vi "MC_7_13a_JW.vi"() -> ()   [LabVIEW 2011]
uses:
  <vilib>/Utility/file.llb/Read From Spreadsheet File (string).vi
  <vilib>/Utility/inputDevices.llb/keyboardAcquire.vi
  <vilib>/Utility/file.llb/Write To Spreadsheet File (DBL).vi
  <vilib>/Utility/file.llb/Write To Spreadsheet File (string).vi
  <vilib>/regexp/Match Regular Expression.xnode
panel:
  out "XY Graph-Lin":cluster{dbl[], dbl[]}[](graph)
  out "Lin Vd":dbl
  out "Lin-Vg Array-Used":dbl[](array[numeric])
  out "Lin Id-Used":dbl[](array[numeric])
  out "Rec: Temp":dbl
  out "Comments":string
  out "Folder Index":dbl caption="Length"
  out "Current \nRecord":string[](array[string])
  out "Transformer \nHeaders":string[](array[string])
  out "Current Device ID":string
  out "Column":string
  out "Row":string
  out "Rec: Concentration":dbl
  out "Rec: Solvent":string
  out "Rec: Method":string
  in  "?":T1(tab)
  out "Rec: Material":string
  in  "Treatment Concentration (mM):":dbl=30.0
  in  "Surface Treatment:":string
  in  "# Drops*:":dbl=inf
  in  "Solution Temp (C):":dbl=55.0
  in  "Relative Humidity (%):":dbl=nan
  in  "Room Temp (F):":dbl=nan
  in  "Time (s):":dbl=80.0
  out "Accel (RPM/s):":dbl
  in  "RPM:":dbl=1000.0
  in  "Wait Time (s):":dbl=10.0
  in  "Sample #:":dbl=1.0
  in  "Fabricator:":string="Jeremy"
  in  "Data File":path
  out "Data Folder":path
  in  "Image Folder":path
  out "Image File":path=path "D:/UserData/Desktop/Jeremy/WFU/Research/Programs/VI mods/Image Not Found.png"
  in  "Ramp (s):":dbl=3.0
  in  "Manuel-Dielectric":bool
  in  "Manuel-Length":bool
  out "Calc: VT-Lin":dbl
  out "New: VT-Lin":dbl
  out "Rec: VT-Lin":dbl caption="VT-Lin" format="%#_3g"
  out "Calc: Trap Density-STS":dbl format="%#_4e"
  out "New: Trap Density-STS":dbl format="%#_4e"
  out "Rec: Trap Density-STS":dbl caption="N-Sat (STS)" format="%#_3e"
  out "Calc: Trap Density-VT":dbl format="%#_4e"
  out "New: Trap Density-VT":dbl format="%#_4e"
  out "Rec: Trap Density-VT":dbl caption="N-Sat (VT)" format="%#_3e"
  out "Calc: Mobility-Lin":dbl format="%#_4e"
  out "New: Mobility-Lin":dbl format="%#_4e"
  out "Rec: Mobility-Lin":dbl caption="Mobility-Lin" format="%#_3e"
  out "Calc: Mobility-Sat":dbl format="%#_4e"
  out "Rec: Length":dbl caption="Length" format="%#_3g"
  out "Rec: Width":dbl caption="Width" format="%#_4g"
  out "Rec: Dielectric (d)":dbl caption="Dielectric (d)" format="%#_3g"
  out "XY Graph":cluster{dbl[], dbl[]}[](graph)
  in  "NumPts":dbl=5.0
  in  "Cancel Button":bool
  in  "Next Button":bool
  in  "Previous Button":bool
  in  "Up Button":bool
  in  "Down Button":bool
  out "Data Name:":string
  in  "Save Changes?":bool
  in  "New: Dielectric":dbl
  in  "New: Length":dbl
  in  "New: Width":dbl
  out "New: Mobility-Sat":dbl format="%#_4e"
  in  "Slide":dbl(slide) step=1.0 scale=-14.3..83.0 scale format="%#_1p"
  in  "Blank Button":bool
  in  "Zoom":i16(slide)=-3 scale=-5.0..5.0
  out "Image Out 2":T2(plugin-control)
  out "Image Out":T2(plugin-control)
  in  "Magnification":u16(ring) items=["5x", "10x", "20x", "50x", "80x"]
  out "Total Width":dbl
  out "Distances":dbl[](array[numeric])
  in  "Undo Button":bool
  in  "Remove Button":bool
  out "Rec: Mobility-Sat":dbl caption="Mobility-Sat" format="%#_3e"
  out "Index":string
  out "Image Name":string
  in  "Export":bool
  out "Calc: VT-Sat":dbl
  out "New: VT-Sat":dbl
  in  "Manual-Width":bool caption="Manual"
  out "XY Graph 2":cluster{dbl[], dbl[]}[](graph)
  in  "Next Button 2":bool
  in  "Previous Button 2":bool
  in  "Slide 2":dbl(slide) step=1.0 scale=-1.0..82.0 scale format="%#_1p"
  out "Calc: STS":dbl
  out "New: STS":dbl
  in  "NumPts 2":dbl=5.0 caption="NumPts"
  out "Rec: VT-Sat":dbl caption="VT-Sat" format="%#_3g"
  out "Rec: STS":dbl caption="STS-Sat" format="%#_3g"
  out "Rec: On/Off":dbl caption="On/Off-Sat" format="%#_3e"
  in  "Save Changes? 2":bool
  in  "Save Changes? 3":bool
  out "Date Recorded":string="Date Recorded" caption="Recorded"
  out "Date Created":string caption="Fabricated"
  out "String":string
  in  "No Image":path=path "D:/UserData/Desktop/Jeremy/WFU/Research/Programs/VI mods/Image Not Found.png"
  in  "Project":path=path "D:/UserData/Desktop/Jeremy/WFU/Research/Programs/Mega Awesome/DeviceData.opj"
  out "Index 2":dbl
  out "Sat Id-Log-Used":dbl[](array[numeric])
  out "Vg Array-Log-Used":dbl[](array[numeric])
  out "ROI Descriptor out":T3 {"Contours"."Type" items=["No Selection", "Point", "Line", "Rectangle", "Oval", "Polygon", "Freehand Region", "Annulus", "Unused2", "Unused3", "Broken Line", "Freehand Line", "Rotated Rectangle"]}
  out "ROI Descriptor":T3 {"Contours"."Type" items=["No Selection", "Point", "Line", "Rectangle", "Oval", "Polygon", "Freehand Region", "Annulus", "Unused2", "Unused3", "Broken Line", "Freehand Line", "Rotated Rectangle"]}
  out "Numeric 3":dbl
  out "Array 6":dbl[][](array[numeric])
  out "Cluster":T4
  out "Array 5":dbl[](array[numeric])
  out "Array 4":dbl[](array[numeric])
  out "Array 3":dbl[](array[numeric])
  out "Numeric 2":dbl
  out "Numeric":dbl
  out "Sat Id-Used":dbl[](array[numeric])
  out "Sat Vg Array-Used":dbl[](array[numeric])
  out "MobVi Index":dbl
  in  "Row Start":dbl=20.0
  # "Data Locations"
  # "Data Location"
  # "Image Location"
  # "Sample Properties"
  # "*     Inf = Full coverage\n   NaN = Unknown or Not Applicable"
  # "Recorded"
  # "Calculated"
  # "Re-Calculated"
  # "Manual"
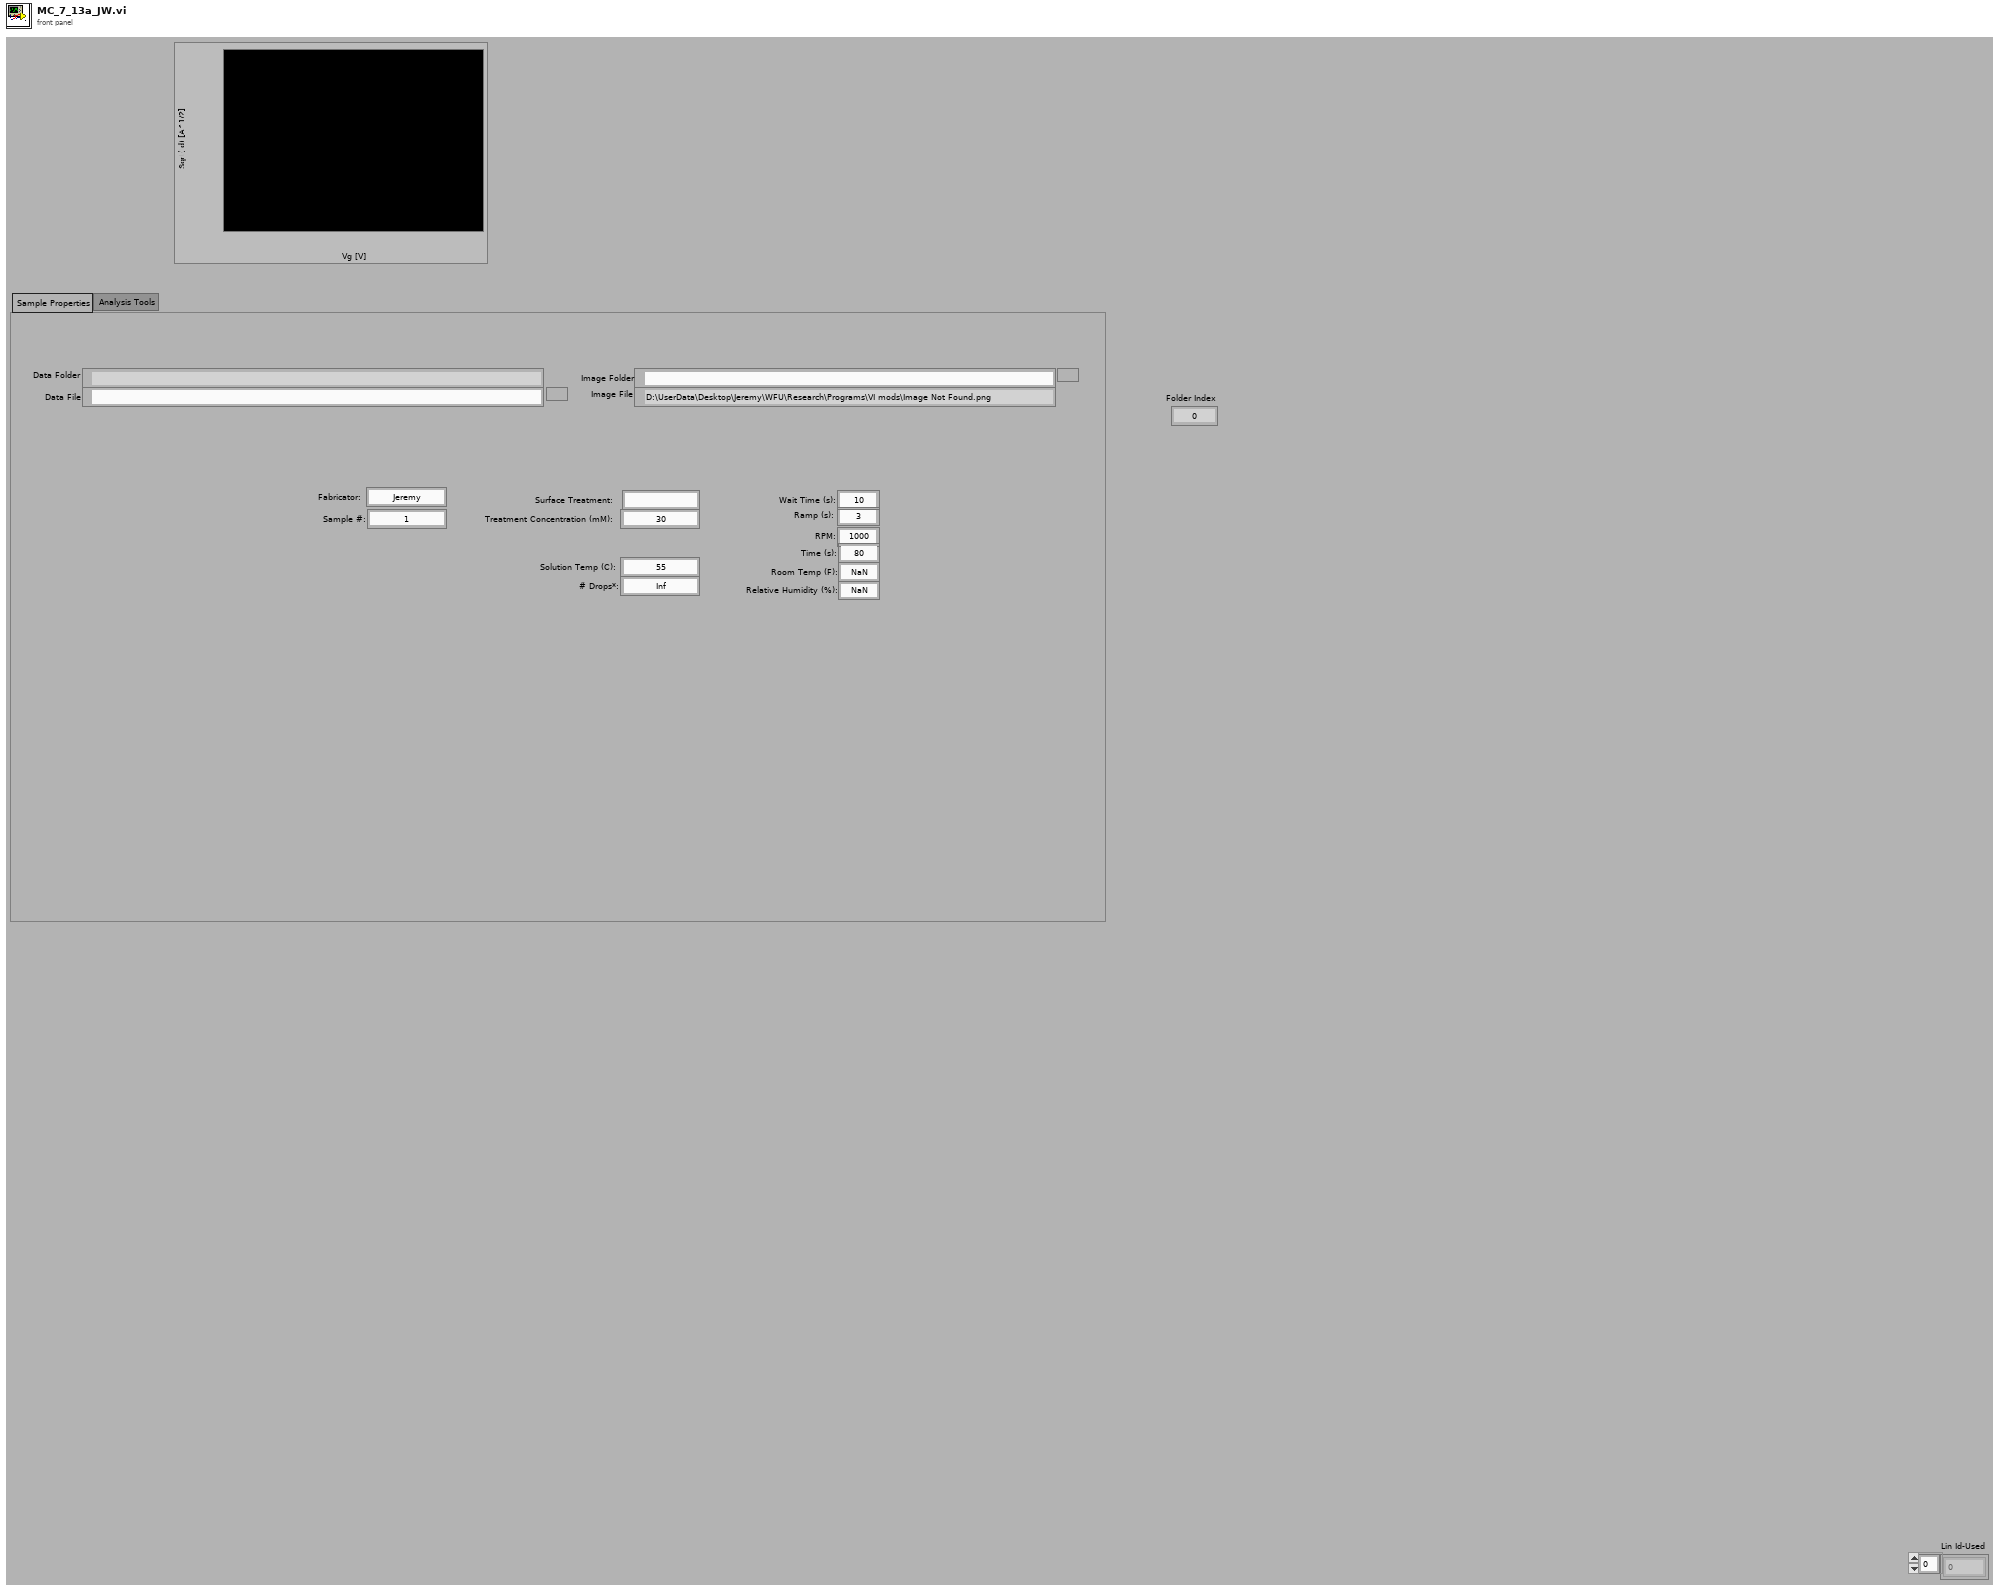
[diagram p1: front panel]
types:
  T1 = enum32{"Sample Properties", "Analysis Tools", "Current Database"}
  T2 = typedef "IMAQ Image.ctl" = refnum<image>
  T3 = typedef "ROI Descriptor" = cluster{"Global Rectangle":i32[], "Contours":cluster{"ID":enum32{"External", "Internal"}, "Type":u32, "Coordinates":i32[]}[]}
  T4 = cluster{"Numeric":dbl, "Numeric 2":dbl, "Numeric 3":dbl, "Numeric 4":dbl}
  T5 = cluster{"Mobility-Sat":dbl, "Moblitity-Lin":dbl, "On/Off":dbl, "Threshold Voltage":dbl, "Onset Voltage":dbl, "STS":dbl, "Trap Density-VT":dbl, "Trap Density-STS":dbl}
  T6 = cluster{"Date Recorded":string, "Index":string, "Length":dbl, "Width":dbl, "Sample Temp":dbl}
  T7 = cluster{"Date Created":string, "Material":string, "Solvent":string, "Concentration":dbl, "Method":string, "Dielectric (nm)":dbl, "Treatment":string, "Comments":string}
  T8 = cluster{"Mobility-Sat":dbl, "Vt-Sat":dbl, "Mobility-Lin":dbl, "Vt-Lin":dbl}
  T9 = cluster{"[0]":cluster{dbl[], dbl[]}, "[1]":cluster{dbl[], dbl[]}, "[2]":cluster{dbl[], dbl[]}, "[3]":cluster{dbl[], dbl[]}, "[4]":cluster{dbl[], dbl[]}, "[5]":cluster{dbl[], dbl[]}, "[6]":cluster{dbl[], dbl[]}, "[7]":cluster{dbl[], dbl[]}, "[8]":cluster{dbl[], dbl[]}}
  T10 = cluster{"Global Rectangle":i32[], "Contours":cluster{"Contour Type":u32, "ROI Type":u32, "Points":i32[]}[]}
  T11 = typedef "LVBoundsTypeDef.ctl" = cluster{"Width":u32, "Height":u32}
  T12 = enum16{"0", "1", "2", "3", "4", "5", "6", "7", "8", "9", "A", "B", "C", "D", "E", "F", "G", "H", "I", "J", "K", "L", "M", "N", "O", "P", "Q", "R", "S", "T", "U", "V", "W", "X", "Y", "Z", "F1", "F2", "F3", "F4", "F5", "F6", "F7", "F8", "F9", "F10", "F11", "F12", "F13", "F14", "F15", "ADD", "BACK", "BACKSLASH", "CAPITAL", "COMMA", "DECIMAL", "DELETE", "DIVIDE", "DOWN", "END", "EQUALS", "ESCAPE", "GRAVE (`)", "HOME", "INSERT", "LBRACKET", "LCONTROL", "LEFT", "L ALT", "LSHIFT", "LWIN", "MINUS", "MULTIPLY", "NEXT", "NUMLOCK", "NUMPAD_0", "NUMPAD_1", "NUMPAD_2", "NUMPAD_3", "NUMPAD_4", "NUMPAD_5", "NUMPAD_6", "NUMPAD_7", "NUMPAD_8", "NUMPAD_9", "PAUSE", "PERIOD", "PRIOR (PG UP)", "RBRACKET", "RCONTROL", "RETURN", "RIGHT", "R ALT", "RSHIFT", "RWIN", "SCROLL", "SEMICOLON", "SLASH", "SPACE", "SUBTRACT", "TAB", "UP", "ENTER (num pad)", "' (quote)"}[]
  T13 = enum16{"0", "1", "2", "3", "4", "5", "6", "7", "8", "9", "A", "B", "C", "D", "E", "F", "G", "H", "I", "J", "K", "L", "M", "N", "O", "P", "Q", "R", "S", "T", "U", "V", "W", "X", "Y", "Z", "F1", "F2", "F3", "F4", "F5", "F6", "F7", "F8", "F9", "F10", "F11", "F12", "F13", "F14", "F15", "ADD", "BACK", "BACKSLASH", "CAPITAL", "COMMA", "DECIMAL", "DELETE", "DIVIDE", "DOWN", "END", "EQUALS", "ESCAPE", "GRAVE (`)", "HOME", "INSERT", "LBRACKET", "LCONTROL", "LEFT", "L ALT", "LSHIFT", "LWIN", "MINUS", "MULTIPLY", "NEXT", "NUMLOCK", "NUMPAD_0", "NUMPAD_1", "NUMPAD_2", "NUMPAD_3", "NUMPAD_4", "NUMPAD_5", "NUMPAD_6", "NUMPAD_7", "NUMPAD_8", "NUMPAD_9", "PAUSE", "PERIOD", "PRIOR (PG UP)", "RBRACKET", "RCONTROL", "RETURN", "RIGHT", "R ALT", "RSHIFT", "RWIN", "SCROLL", "SEMICOLON", "SLASH", "SPACE", "SUBTRACT", "TAB", "UP", "ENTER (num pad)", "' (quote)"}
  T14 = cluster{"Contour Type":u32, "ROI Type":u32, "Points":i32[]}[]
  T15 = cluster{i32[], cluster{"Contour Type":u32, "ROI Type":u32, "Points":i32[]}[]}
  T16 = cluster{string, sgl, bool, bool, bool, bool, bool, bool, i32}
  T17 = cluster{i32, cluster{string, sgl, bool, bool, bool, bool, bool, bool, i32}, i32, i32}
  T18 = cluster{"Contour Type":u32, "ROI Type":u32, "Points":i32[]}
  T19 = cluster{"Points[0]":i32, "Points[1]":i32, "Points[2]":i32, "Points[3]":i32, "Points[4]":i32, "Points[5]":i32, "Points[6]":i32, "Points[7]":i32, "Points[8]":i32}
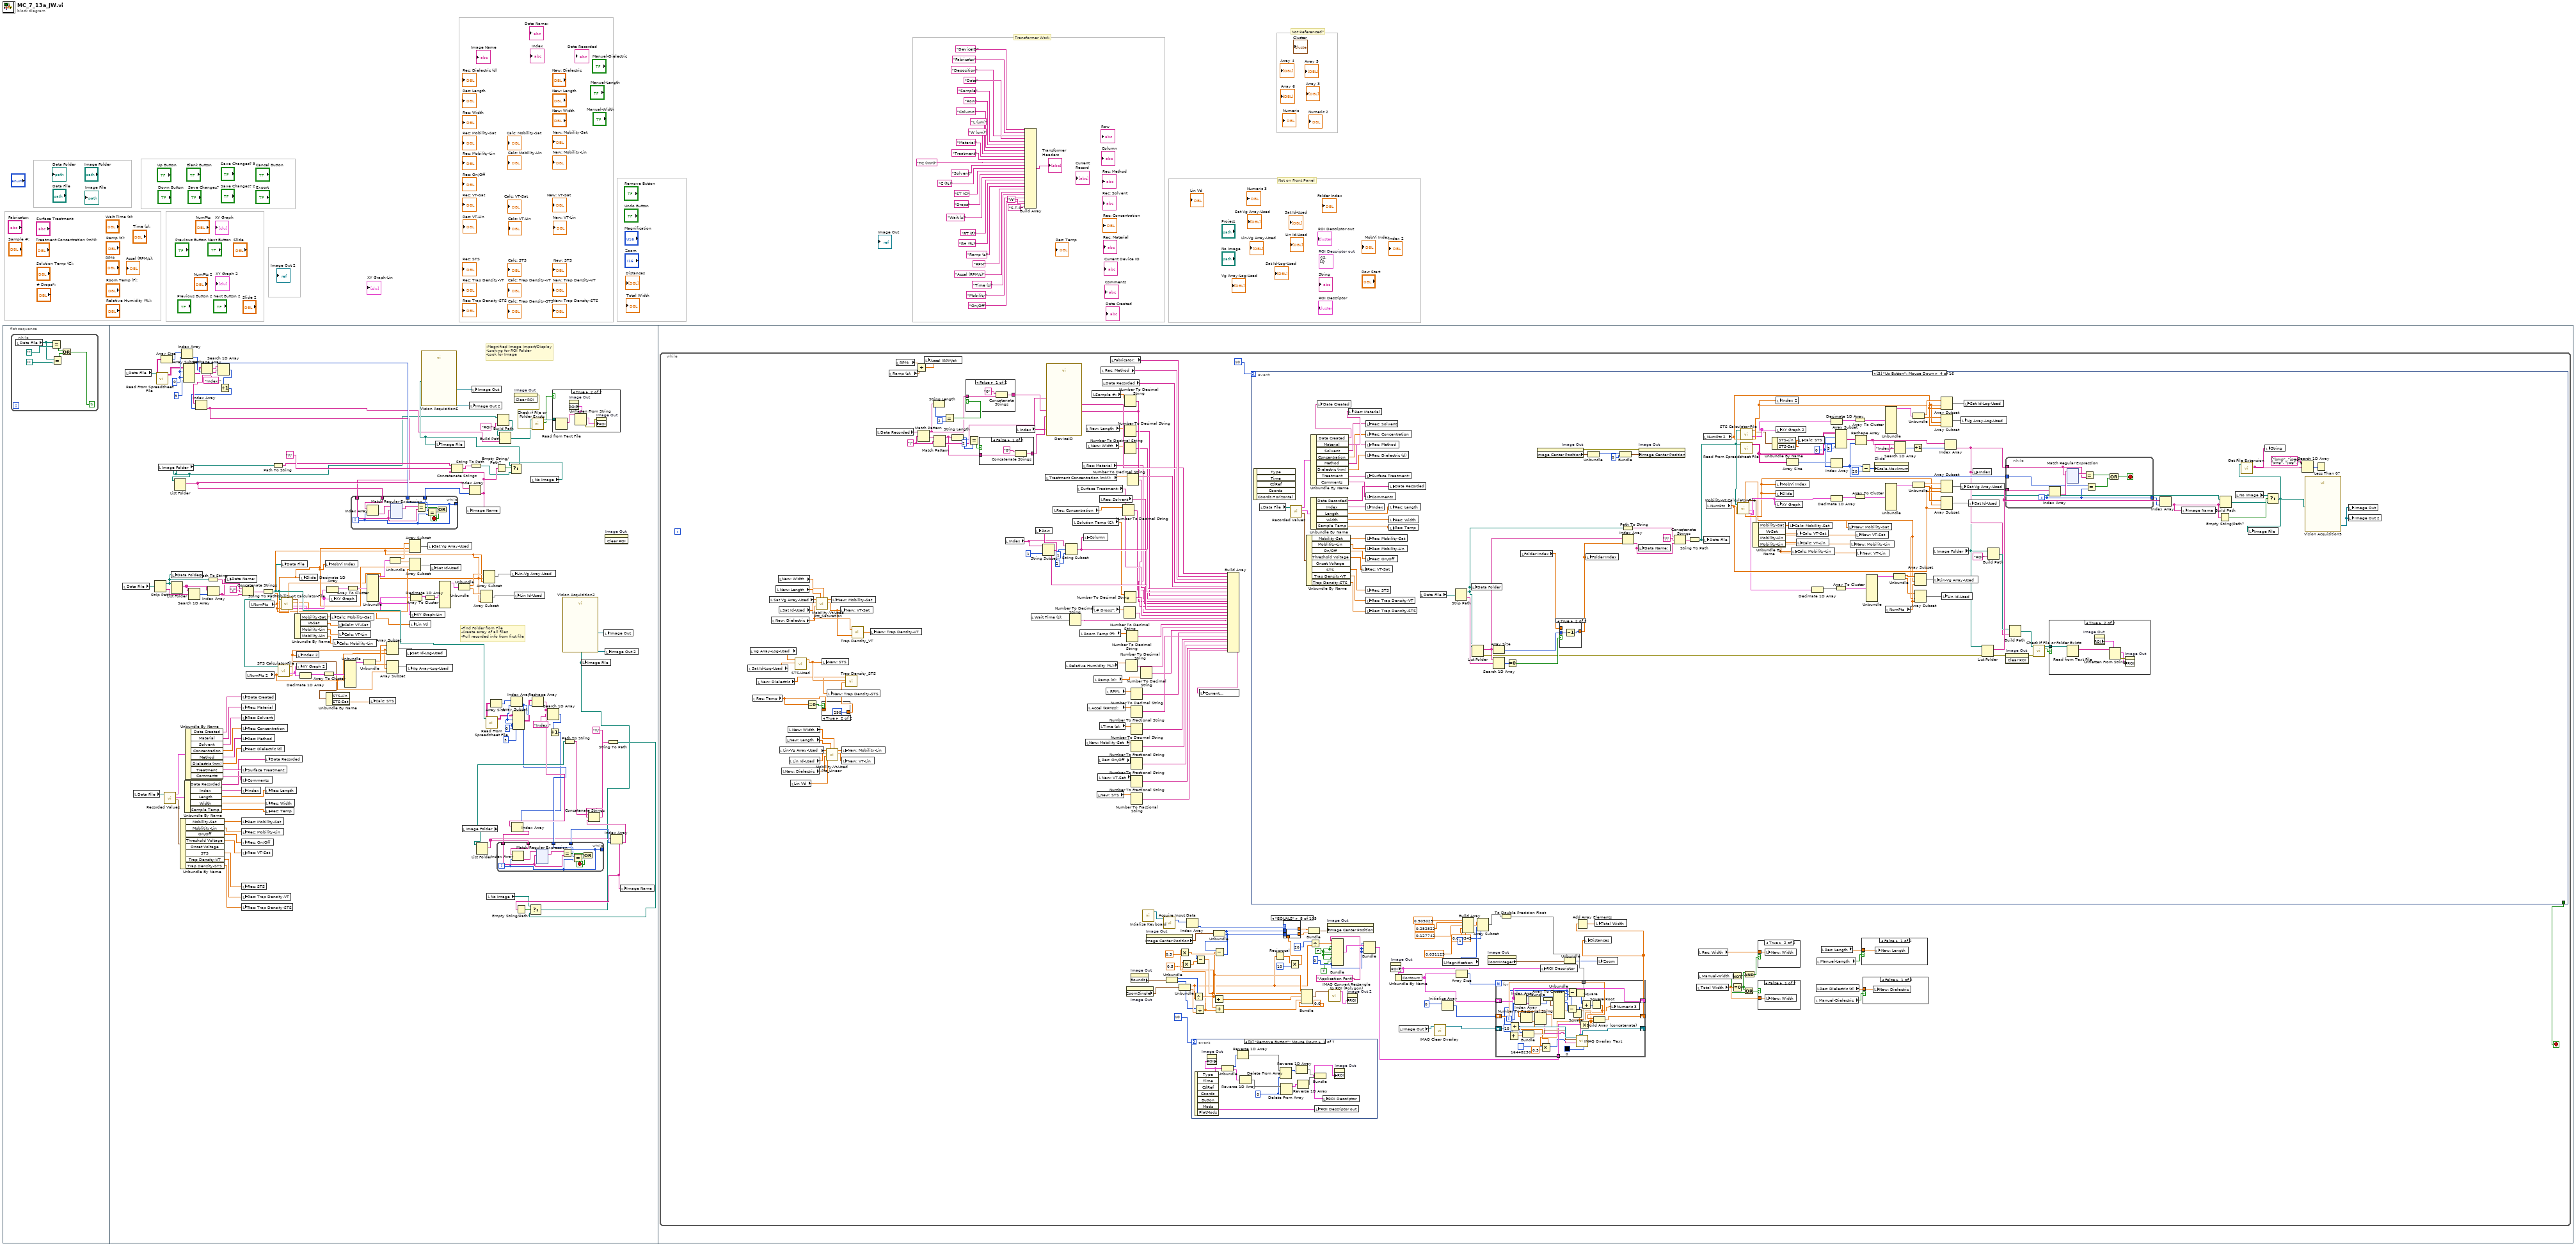
[diagram p0: block diagram]
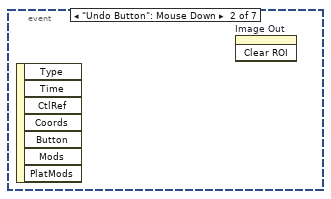
[diagram p10: hidden frame]
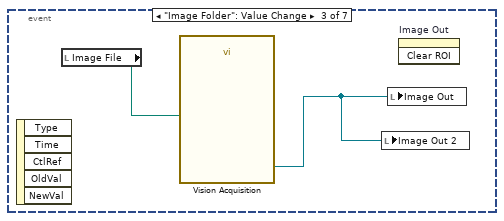
[diagram p11: hidden frame]
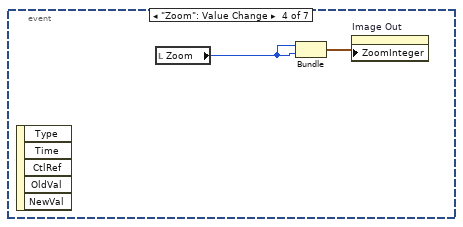
[diagram p12: hidden frame]
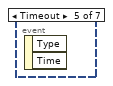
[diagram p13: hidden frame]
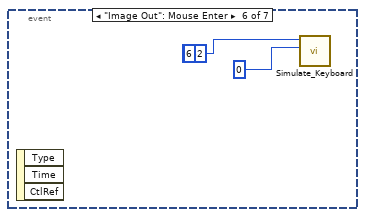
[diagram p14: hidden frame]
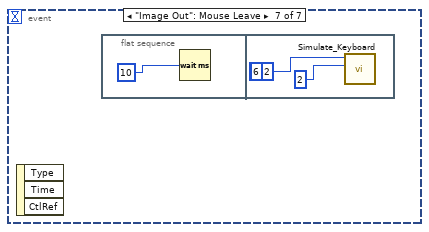
[diagram p15: hidden frame]
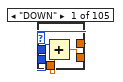
[diagram p16: hidden frame]
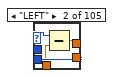
[diagram p17: hidden frame]
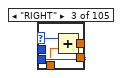
[diagram p18: hidden frame]
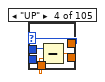
[diagram p19: hidden frame]
diagram:
  (unwired) T3 {"Global Rectangle"=[], "Contours"=[]}  # ROI Descriptor out
  # "Not Referenced?"
  # "Transformer Work"
  # "Not on Front Panel"
  n1 = flat-sequence {
    frame #0 {
      n2 = while {
        stop <- w29 continue-if-true
        n3 = local read "Data File"() -> (w31:path)
        n4 = Equal?(x=w31, y=path "") -> (x = y?=w33:bool)
        n5 = Equal?(x=w31, y=path "") -> (x = y?=w32:bool)
        n6 = Or(x=w33, y=w32) -> (x .or. y?=w29:bool)
      }
    }
    frame #1 {
      w123 = 0
      w147 = 0
      # "-Find Folder from File\n-Create array of all files\n-Pull recorded info from first file"
      # "-Magnified Image Import/Display\n-Looking for ROI Folder\n-Look for Image"
      n7 = local read "Data File"() -> (w127:path)
      n8 = local read "Data File"() -> (w142:path)
      n9 = local read "Data File"() -> (w82:path)
      n10 = Strip Path(path=w127) -> (stripped path=w128:path, name=w114:string)
      n11 = call-poly <vilib>:"Read From Spreadsheet File.vi"("file path (dialog if empty)"=w142) -> ("all rows"=w145:string[][])  [unwired: 6 in, 4 out]
      n12 = local read "Image Folder"() -> (w84:path)
      n13 = Array Size(array=w145) -> (size(s)=w146:i32[])
      n14 = call "Recorded Values.vi"("Path"=w82) -> ("Recorded Char"=w80:T5, "Recorded Prop"=w79:T6, "Fabrication Prop"=w81:T7)  [unwired: 8 in]
      n15 = local write "Data Folder"(w128) -> ()
      n16 = List Folder(path=w128) -> (filenames=w118:string[])  [unwired: 3 in, 3 out]
      n17 = List Folder(path=w84) -> (filenames=w151:string[])  [unwired: 3 in, 3 out]
      n18 = Unbundle By Name(w80) -> ("Mobility-Sat"=w66:dbl, "Moblitity-Lin"=w65:dbl, "On/Off"=w64:dbl, "Threshold Voltage"=w63:dbl, "STS"=w62:dbl, "Trap Density-VT"=w61:dbl, "Trap Density-STS"=w60:dbl)  [unwired: 1 out]
      n19 = Index Array(array=w146, index=w147) -> (element=w153:i32)
      n20 = Array Subset(array=w145, index (row)=w147, index (col)=w147, length (col)=3) -> (w144:string[][])  [unwired: 1 in]
      n21 = Unbundle By Name(w79) -> ("Date Recorded"=w71:string, "Index"=w70:string, "Length"=w69:dbl, "Width"=w68:dbl, "Sample Temp"=w67:dbl)
      n22 = Unbundle By Name(w81) -> ("Date Created"=w59:string, "Material"=w78:string, "Solvent"=w77:string, "Concentration"=w76:dbl, "Method"=w75:string, "Dielectric (nm)"=w74:dbl, "Treatment"=w73:string, "Comments"=w72:string)
      n23 = Search 1D Array(1D array=w118, element=w114) -> (index of element=w117:i32)  [unwired: 1 in]
      n24 = Reshape Array(w144, w153) -> (w158:string[])
      n25 = Path To String(path=w128) -> (string=w113:string)
      n26 = Index Array(array=w118, index=w117) -> (element=w83:string)
      n27 = Search 1D Array(1D array=w158, element="Index:") -> (index of element=w150:i32)  [unwired: 1 in]
      n28 = Increment(x=w150) -> (x+1=w149:i32)
      n29 = Index Array(array=w158, index=w149) -> (element=w85:string)
      n30 = local write "Data Name:"(w83) -> ()
      n31 = local write "Date Created"(w59) -> ()
      n32 = local write "Rec: Material"(w78) -> ()
      n33 = local write "Rec: Solvent"(w77) -> ()
      n34 = local write "Rec: Concentration"(w76) -> ()
      n35 = local write "Rec: Method"(w75) -> ()
      n36 = local write "Rec: Dielectric (d)"(w74) -> ()
      n37 = local write "Surface Treatment:"(w73) -> ()
      n38 = local write "Comments"(w72) -> ()
      n39 = local write "Index"(w70) -> ()
      n40 = local write "Rec: Mobility-Sat"(w66) -> ()
      n41 = local write "Rec: Mobility-Lin"(w65) -> ()
      n42 = local write "Rec: On/Off"(w64) -> ()
      n43 = local write "Rec: VT-Sat"(w63) -> ()
      n44 = local write "Rec: STS"(w62) -> ()
      n45 = local write "Rec: Trap Density-VT"(w61) -> ()
      n46 = local write "Rec: Trap Density-STS"(w60) -> ()
      n47 = Concatenate Strings(w113, "\\", w83) -> (w115:string)
      n48 = local read "NumPts 2"() -> (w50:dbl)
      n49 = local read "NumPts"() -> (w40:dbl)
      n50 = String To Path(string=w115) -> (path=w58:path)
      n51 = local write "Date Recorded"(w71) -> ()
      n52 = local write "Rec: Length"(w69) -> ()
      n53 = local write "Rec: Width"(w68) -> ()
      n54 = local write "Rec: Temp"(w67) -> ()
      n55 = Path To String(path=w84) -> (string=w155:string)
      n56 = call "STS Calculator-File.vi"("NumPts"=w50, "Path"=w58) -> ("STS Index-Sat"=w48:dbl, "XY Graph-Sat"=w49:cluster{dbl[], dbl[]}[], "Ouput"=w47:cluster{"STS-Sat":dbl, "STS-Lin":dbl})  [unwired: 5 in, 2 out]
      n57 = local write "Data File"(w58) -> ()
      n58 = call "Mobility-Vt Calculator-File.vi"("NumPts"=w40, "Path"=w58) -> ("XY Graph-Sat"=w52:cluster{dbl[], dbl[]}[], "XY Graph-Lin"=w35:cluster{dbl[], dbl[]}[], "Lin Vd"=w36:dbl, "Output"=w53:T8, "Index-Sat"=w51:dbl, "Index-Lin"=w39:dbl)  [unwired: 4 in]
      n59 = Unbundle By Name(w53) -> ("Mobility-Sat"=w57:dbl, "Vt-Sat"=w56:dbl, "Mobility-Lin"=w55:dbl, "Mobility-Lin"=w54:dbl)
      n60 = local write "Index 2"(w48) -> ()
      n61 = local write "XY Graph 2"(w49) -> ()
      n62 = local write "Slide"(w51) -> ()
      n63 = Decimate 1D Array(w49) -> (w105:cluster{dbl[], dbl[]}[])  [unwired: 1 out]
      n64 = Array To Cluster(array=w105) -> (cluster=w107:T9)
      n65 = local write "MobVi Index"(w51) -> ()
      n66 = Unbundle By Name(w47) -> ("STS-Sat"=w46:dbl)  [unwired: 1 out]
      n67 = Decimate 1D Array(w52) -> (w141:cluster{dbl[], dbl[]}[])  [unwired: 1 out]
      n68 = local write "XY Graph"(w52) -> ()
      n69 = local write "Calc: Mobility-Sat"(w57) -> ()
      n70 = local write "Calc: Mobility-Lin"(w54) -> ()
      n71 = local write "Calc: VT-Sat"(w56) -> ()
      n72 = local write "Calc: VT-Lin"(w55) -> ()
      n73 = Unbundle(w107) -> ("[0]"=w106:cluster{dbl[], dbl[]})  [unwired: 8 out]
      n74 = Array To Cluster(array=w141) -> (cluster=w139:T9)
      n75 = while {
        tunnel: w151 -> [w291]
        tunnel: w85 -> [w289]
        tunnel: [w288] -> _
        tunnel: [w288] -> w152
        tunnel: w153 -> [w287]
        i -> [w288]
        stop <- w284 stop-if-true
        n76 = Index Array(array=w291, index=w288) -> (element=w292:string)
        n77 = xnode "Match Regular Expression"("input string"=w292, "regular expression"=w289) -> ("whole match"=w290:string)  [unwired: 4 in, 4 out]
        n78 = Equal?(x=w290, y=w289) -> (x = y?=w286:bool)
        n79 = Equal?(x=w287, y=w288) -> (x = y?=w285:bool)
        n80 = Or(x=w286, y=w285) -> (x .or. y?=w284:bool)
      }
      n81 = Unbundle(w106) -> (w103:dbl[], w102:dbl[])
      n82 = Unbundle(w139) -> ("[0]"=w140:cluster{dbl[], dbl[]})  [unwired: 8 out]
      n83 = local write "Calc: STS"(w46) -> ()
      n84 = Array Subset(array=w103, index=w48, length=w50) -> (w110:dbl[])
      n85 = Array Subset(array=w102, index=w48, length=w50) -> (w109:dbl[])
      n86 = Unbundle(w140) -> (w104:dbl[], w108:dbl[])
      n87 = local write "Sat Id-Log-Used"(w110) -> ()
      n88 = local write "Vg Array-Log-Used"(w109) -> ()
      n89 = Array Subset(array=w104, index=w51, length=w40) -> (w111:dbl[])
      n90 = Array Subset(array=w108, index=w51, length=w40) -> (w112:dbl[])
      n91 = local write "Lin Vd"(w36) -> ()
      n92 = Decimate 1D Array(w35) -> (w45:cluster{dbl[], dbl[]}[])  [unwired: 1 out]
      n93 = local write "XY Graph-Lin"(w35) -> ()
      n94 = Array To Cluster(array=w45) -> (cluster=w44:T9)
      n95 = local write "Sat Vg Array-Used"(w111) -> ()
      n96 = local write "Sat Id-Used"(w112) -> ()
      n97 = Unbundle(w44) -> ("[0]"=w43:cluster{dbl[], dbl[]})  [unwired: 8 out]
      n98 = Unbundle(w43) -> (w42:dbl[], w41:dbl[])
      n99 = local read "Image Folder"() -> (w134:path)
      n100 = Index Array(array=w151, index=w152) -> (element=w101:string)
      n101 = Concatenate Strings(w155, "\\", w101) -> (w156:string)
      n102 = local write "Image Name"(w101) -> ()
      n103 = String To Path(string=w156) -> (path=w99:path)
      n104 = List Folder(path=w134) -> (filenames=w130:string[])  [unwired: 3 in, 3 out]
      n105 = Array Subset(array=w41, index=w39, length=w40) -> (w37:dbl[])
      n106 = Array Subset(array=w42, index=w39, length=w40) -> (w38:dbl[])
      n107 = call-poly <vilib>:"Read From Spreadsheet File.vi"("file path (dialog if empty)"=w58) -> ("all rows"=w121:string[][])  [unwired: 6 in, 4 out]
      n108 = local read "No Image"() -> (w93:path)
      n109 = Array Size(array=w121) -> (size(s)=w122:i32[])
      n110 = Empty String/Path?(string/path=w101) -> (empty?=w100:bool)
      n111 = Build Path(base path=w84, name or relative path="ROI") -> (appended path=w87:path)
      n112 = Build Path(base path=w87, name or relative path=w85) -> (appended path=w86:path)
      n113 = Index Array(array=w122, index=w123) -> (element=w133:i32)
      n114 = local write "Lin-Vg Array-Used"(w38) -> ()
      n115 = Array Subset(array=w121, index (row)=w123, index (col)=w123, length (col)=3) -> (w120:string[][])  [unwired: 1 in]
      n116 = local write "Lin Id-Used"(w37) -> ()
      n117 = invoke on="Image Out" class="ImageControl" method="Clear ROI"() -> (error out=w91:errorcluster)  [unwired: 3 in, 2 out]
      n118 = local read "No Image"() -> (w92:path)
      n119 = Select(t=w92, s=w100, f=w99) -> (s? t:f=w98:path)
      n120 = call "Vision Acquisition6"("Image Path"=w98) -> ("Image Out"=w154:T2)  [unwired: 25 in, 1 out]
      n121 = local write "Image File"(w98) -> ()
      n122 = local write "Image Out 2"(w154) -> ()
      n123 = local write "Image Out"(w154) -> ()
      n124 = call <vilib>:"Check if File or Folder Exists.vi"("error in (no error)"=w91, "path"=w86) -> ("file or folder exists?"=w89:bool, "dup path"=w90:path)  [unwired: 7 in, 1 out]
      n125 = Reshape Array(w120, w133) -> (w138:string[])
      n126 = Search 1D Array(1D array=w138, element="Index:") -> (index of element=w126:i32)  [unwired: 1 in]
      n127 = Increment(x=w126) -> (x+1=w125:i32)
      n128 = Index Array(array=w138, index=w125) -> (element=w131:string)
      n129 = while {
        tunnel: w130 -> [w171]
        tunnel: w131 -> [w169]
        tunnel: [w168] -> _
        tunnel: [w168] -> w132
        tunnel: w133 -> [w167]
        i -> [w168]
        stop <- w164 stop-if-true
        n130 = Index Array(array=w171, index=w168) -> (element=w172:string)
        n131 = xnode "Match Regular Expression"("input string"=w172, "regular expression"=w169) -> ("whole match"=w170:string)  [unwired: 4 in, 4 out]
        n132 = Equal?(x=w170, y=w169) -> (x = y?=w166:bool)
        n133 = Equal?(x=w167, y=w168) -> (x = y?=w165:bool)
        n134 = Or(x=w166, y=w165) -> (x .or. y?=w164:bool)
      }
      n135 = case shown="True" w89 {
        tunnel: w90 -> [_ w159]
        frame False {
        }
        frame True {
          n136 = Read from Text File(file (use dialog)=w159) -> (text=w163:string)  [unwired: 3 in, 3 out]
          n137 = property on="Image Out" class="ImageControl"() -> ("ROI"=w160:T10)  [unwired: 2 in, 2 out]
          n138 = Unflatten From String(type=w160, binary string=w163) -> (value=w161:T10, error out=w162:errorcluster)  [unwired: 3 in, 1 out]
          n139 = property on="Image Out" class="ImageControl"(error in=w162, "ROI"=w161) -> ()  [unwired: 1 in, 2 out]
        }
      }
      n140 = Path To String(path=w134) -> (string=w135:string)
      n141 = invoke on="Image Out" class="ImageControl" method="Clear ROI"() -> ()  [unwired: 3 in, 3 out]
      n142 = Index Array(array=w130, index=w132) -> (element=w96:string)
      n143 = Empty String/Path?(string/path=w96) -> (empty?=w97:bool)
      n144 = Concatenate Strings(w135, "\\", w96) -> (w136:string)
      n145 = String To Path(string=w136) -> (path=w95:path)
      n146 = Select(t=w93, s=w97, f=w95) -> (s? t:f=w94:path)
      n147 = call "Vision Acquisition2"("Image Path"=w94) -> ("Image Out"=w129:T2)  [unwired: 25 in, 1 out]
      n148 = local write "Image File"(w94) -> ()
      n149 = local write "Image Out"(w129) -> ()
      n150 = local write "Image Out 2"(w129) -> ()
      n151 = local write "Image Name"(w96) -> ()
    }
    frame #2 {
      n152 = while {
        stop <- w569 stop-if-true
        w465 = "/"
        w519 = FALSE
        w517 = 0
        n153 = local read "Sat Id-Log-Used"() -> (w422:dbl[])
        n154 = local read "Vg Array-Log-Used"() -> (w421:dbl[])
        n155 = local read "Rec: Temp"() -> (w411:dbl)
        n156 = local read "New: Dielectric"() -> (w408:dbl)
        n157 = local read "Sat Vg Array-Used"() -> (w424:dbl[])
        n158 = local read "New: Dielectric"() -> (w405:dbl)
        n159 = local read "New: Length"() -> (w425:dbl)
        n160 = local read "New: Width"() -> (w427:dbl)
        n161 = local read "Sat Id-Used"() -> (w423:dbl[])
        n162 = local read "Lin-Vg Array-Used"() -> (w418:dbl[])
        n163 = local read "New: Dielectric"() -> (w415:dbl)
        n164 = local read "New: Length"() -> (w417:dbl)
        n165 = local read "New: Width"() -> (w414:dbl)
        n166 = local read "Lin Id-Used"() -> (w419:dbl[])
        n167 = local read "Lin Vd"() -> (w413:dbl)
        n168 = call "STS-Used.vi"("Id Used"=w422, "Vg-Used"=w421) -> ("STS"=w412:dbl)  [unwired: 9 in]
        n169 = Equal To 0?(x=w411) -> (x = 0?=w410:bool)
        n170 = call "Mobility-Vt-Used Pts_Saturation.vi"("Width"=w427, "Length"=w425, "Dielectric (d)"=w405, "Sat Id Used"=w423, "Vg Used"=w424) -> ("Vt"=w406:dbl, "Mobility"=w426:dbl)  [unwired: 4 in, 1 out]
        n171 = local write "New: STS"(w412) -> ()
        n172 = case shown="True" w410 {
          tunnel: [w570 290] -> w409
          tunnel: w411 -> [w570 _]
          frame False {
          }
          frame True {
          }
        }
        n173 = call "Mobility-Vt-Used Pts_Linear.vi"("Width"=w414, "Length"=w417, "Vd"=w413, "Dielectric (d)"=w415, "Sat Id Used"=w419, "Vg Used"=w418) -> ("Vt"=w420:dbl, "Mobility"=w416:dbl)  [unwired: 3 in, 1 out]
        n174 = local write "New: Mobility-Sat"(w426) -> ()
        n175 = local write "New: VT-Sat"(w406) -> ()
        n176 = local write "New: Mobility-Lin"(w416) -> ()
        n177 = local write "New: VT-Lin"(w420) -> ()
        n178 = call "Trap Density_STS.vi"("Temp (T) [K]"=w409, "S.T.S. (S)"=w412, "Dielectric"=w408) -> ("Trap Density (N)"=w407:dbl)  [unwired: 8 in]
        n179 = local write "New: Trap Density-STS"(w407) -> ()
        n180 = call "Trap Density_VT.vi"("VT"=w406, "Dielectric"=w405) -> ("Trap Density-VT"=w404:dbl)
        n181 = local write "New: Trap Density-VT"(w404) -> ()
        n182 = local read "Date Recorded"() -> (w468:string)
        n183 = local read "Ramp (s):"() -> (w435:dbl)
        n184 = local read "RPM:"() -> (w436:dbl)
        n185 = Divide(x=w436, y=w435) -> (x/y=w434:dbl)
        n186 = Match Pattern(string=w468, regular expression=w465) -> (before substring=w459:string, after substring=w466:string)  [unwired: 1 in, 2 out]
        n187 = local write "Accel (RPM/s):"(w434) -> ()
        n188 = String Length(string=w459) -> (length=w462:i32)
        n189 = Match Pattern(string=w466, regular expression=w465) -> (before substring=w453:string, after substring=w464:string)  [unwired: 1 in, 2 out]
        n190 = Equal?(x=w462, y=2) -> (x = y?=w460:bool)
        n191 = String Length(string=w453) -> (length=w455:i32)
        n192 = case shown="False" w460 {
          tunnel: w459 -> [w579 w581]
          tunnel: [w578 w581] -> w458
          frame False {
            n193 = Concatenate Strings("0", w579) -> (w578:string)
          }
          frame True {
          }
        }
        n194 = Equal?(x=w455, y=2) -> (x = y?=w457:bool)
        n195 = case shown="False" w457 {
          tunnel: w453 -> [w575 w577]
          tunnel: [w574 w577] -> w454
          frame False {
            n196 = Concatenate Strings("0", w575) -> (w574:string)
          }
          frame True {
          }
        }
        n197 = local read "Index"() -> (w438:string)
        n198 = local read "Index"() -> (w452:string)
        n199 = local read "Wait Time (s):"() -> (w498:dbl)
        n200 = String Subset(string=w438, length (rest)=1) -> (substring=w493:string)  [unwired: 1 in]
        n201 = local write "Row"(w493) -> ()
        n202 = local read "Treatment Concentration (mM):"() -> (w446:dbl)
        n203 = local read "Rec: Concentration"() -> (w433:dbl)
        n204 = local read "Relative Humidity (%):"() -> (w443:dbl)
        n205 = String Subset(string=w438, offset (0)=1, length (rest)=2) -> (substring=w494:string)
        n206 = Number To Decimal String(number=w498) -> (decimal integer string=w499:string)  [unwired: 1 in]
        n207 = local read "Solution Temp (C):"() -> (w487:dbl)
        n208 = local read "Surface Treatment:"() -> (w445:string)
        n209 = local read "Room Temp (F):"() -> (w491:dbl)
        n210 = local read "Rec: Material"() -> (w441:string)
        n211 = local write "Column"(w494) -> ()
        n212 = local read "New: Mobility-Sat"() -> (w480:dbl)
        n213 = local read "New: Length"() -> (w451:dbl)
        n214 = local read "New: Width"() -> (w450:dbl)
        n215 = local read "Accel (RPM/s):"() -> (w478:dbl)
        n216 = local read "Sample #:"() -> (w470:dbl)
        n217 = local read "# Drops*:"() -> (w488:dbl)
        n218 = local read "Ramp (s):"() -> (w496:dbl)
        n219 = local read "New: STS"() -> (w472:dbl)
        n220 = local read "New: VT-Sat"() -> (w474:dbl)
        n221 = local read "Rec: On/Off"() -> (w476:dbl)
        n222 = local read "Rec: Solvent"() -> (w447:string)
        n223 = local read "Time (s):"() -> (w483:dbl)
        n224 = local read "Rec: Method"() -> (w471:string)
        n225 = local read "Date Recorded"() -> (w467:string)
        n226 = local read "RPM:"() -> (w484:dbl)
        n227 = local read "Fabricator:"() -> (w492:string)
        n228 = Number To Decimal String(number=w433) -> (decimal integer string=w432:string)  [unwired: 1 in]
        n229 = Number To Decimal String(number=w488) -> (decimal integer string=w489:string)  [unwired: 1 in]
        n230 = Number To Decimal String(number=w470) -> (decimal integer string=w463:string)  [unwired: 1 in]
        n231 = call "DeviceID"("Sample"=w463, "Year"=w464, "Month"=w458, "Day"=w454, "Index"=w452) -> ("Result"=w469:string)  [unwired: 9 in, 1 out]
        n232 = Number To Decimal String(number=w451) -> (decimal integer string=w449:string)  [unwired: 1 in]
        n233 = Number To Decimal String(number=w450) -> (decimal integer string=w448:string)  [unwired: 1 in]
        n234 = Number To Decimal String(number=w487) -> (decimal integer string=w486:string)  [unwired: 1 in]
        n235 = Number To Decimal String(number=w443) -> (decimal integer string=w442:string)  [unwired: 1 in]
        n236 = Number To Decimal String(number=w491) -> (decimal integer string=w490:string)  [unwired: 1 in]
        n237 = property on="Image Out" class="ImageControl"() -> ("ZoomSingle"=w537:cluster{"X":sgl, "Y":sgl})  [unwired: 2 in, 2 out]
        n238 = Number To Decimal String(number=w446) -> (decimal integer string=w444:string)  [unwired: 1 in]
        n239 = property on="Image Out" class="ImageControl"() -> ("Bounds"=w538:T11)  [unwired: 2 in, 2 out]
        n240 = Number To Decimal String(number=w484) -> (decimal integer string=w485:string)  [unwired: 1 in]
        n241 = Number To Fractional String(number=w478) -> (F-format string=w479:string)  [unwired: 3 in]
        n242 = Number To Decimal String(number=w483) -> (decimal integer string=w482:string)  [unwired: 1 in]
        n243 = Number To Fractional String(number=w480) -> (F-format string=w481:string)  [unwired: 3 in]
        n244 = Number To Fractional String(number=w476) -> (F-format string=w477:string)  [unwired: 3 in]
        n245 = Number To Fractional String(number=w474) -> (F-format string=w475:string)  [unwired: 3 in]
        n246 = Number To Fractional String(number=w472) -> (F-format string=w473:string)  [unwired: 3 in]
        n247 = Number To Decimal String(number=w496) -> (decimal integer string=w497:string)  [unwired: 1 in]
        n248 = call <vilib>:"Intialize Keyboard.vi"() -> ("device ID"=w549:refnum<k1>)  [unwired: 10 in, 1 out]
        n249 = property on="Image Out" class="ImageControl"() -> ("Image Center Position"=w544:cluster{"X":u32, "Y":u32})  [unwired: 2 in, 2 out]
        n250 = call-poly <vilib>:"Acquire Input Data.vi"("device ID"=w549) -> ("keys pressed"=w548:T12)  [unwired: 16 in, 2 out]
        n251 = Unbundle(w538) -> ("Width"=w535:u32, "Height"=w534:u32)
        n252 = Unbundle(w537) -> ("X"=w512:sgl, "Y"=w536:sgl)
        n253 = Index Array(array=w548) -> (element=w552:T13)  [unwired: 1 in]
        n254 = event shown="[0] \"Remove Button\": Mouse Down" {
          selector: _ -> [_ _ _ _ _ _ _]
          dyn-events: _ -> [_ _ _ _ _ _ _]
          timeout: 10 -> [_ _ _ _ _ _ _]
          event "Remove Button": Mouse Down {
            w586 = 0
            n255 = event-data() -> ()  [unwired: 1 in, 7 out]
            n256 = property on="Image Out" class="ImageControl"() -> ("ROI"=w584:T10)  [unwired: 2 in, 2 out]
            n257 = Unbundle(w584) -> ("Global Rectangle"=w587:i32[], "Contours"=w589:T14)
            n258 = Reverse 1D Array(array=w587) -> (reversed array=w588:i32[])
            n259 = Reverse 1D Array(array=w589) -> (reversed array=w590:T14)
            n260 = Delete From Array(array=w588, index=w586) -> (array with subset deleted=w591:i32[])  [unwired: 1 in, 1 out]
            n261 = Delete From Array(array=w590, index=w586) -> (array with subset deleted=w592:T14)  [unwired: 1 in, 1 out]
            n262 = Reverse 1D Array(array=w591) -> (reversed array=w593:i32[])
            n263 = Reverse 1D Array(array=w592) -> (reversed array=w594:T14)
            n264 = Bundle(w593, w594) -> (w585:T15)  [unwired: 1 in]
            n265 = local write "ROI Descriptor out"(w584) -> ()
            n266 = local write "ROI Descriptor"(w585) -> ()
            n267 = property on="Image Out" class="ImageControl"("ROI"=w585) -> ()  [unwired: 2 in, 2 out]
          }
          event "Undo Button": Mouse Down {
            n268 = event-data() -> ()  [unwired: 1 in, 7 out]
            n269 = invoke on="Image Out" class="ImageControl" method="Clear ROI"() -> ()  [unwired: 3 in, 3 out]
          }
          event "Image Folder": Value Change {
            n270 = event-data() -> ()  [unwired: 1 in, 5 out]
            n271 = local read "Image File"() -> (w596:path)
            n272 = call "Vision Acquisition"("Image Path"=w596) -> ("Image Out"=w595:T2)  [unwired: 25 in, 1 out]
            n273 = local write "Image Out 2"(w595) -> ()
            n274 = local write "Image Out"(w595) -> ()
            n275 = invoke on="Image Out" class="ImageControl" method="Clear ROI"() -> ()  [unwired: 3 in, 3 out]
          }
          event "Zoom": Value Change {
            n276 = event-data() -> ()  [unwired: 1 in, 5 out]
            n277 = local read "Zoom"() -> (w597:i16)
            n278 = Bundle("Zoom"=w597, "Zoom"=w597) -> (w598:cluster{"Zoom":i16, "Zoom":i16})  [unwired: 1 in]
            n279 = property on="Image Out" class="ImageControl"("ZoomInteger"=w598) -> ()  [unwired: 2 in, 2 out]
          }
          event Timeout {
            n280 = event-data() -> ()  [unwired: 1 in, 2 out]
          }
          event "Image Out": Mouse Enter {
            (unwired) 6
            n281 = event-data() -> ()  [unwired: 1 in, 3 out]
            n282 = call "Simulate_Keyboard.vi"("Action"=0, "Virtual Key"=162) -> ()  [unwired: 7 in, 1 out]
          }
          event "Image Out": Mouse Leave {
            n283 = event-data() -> ()  [unwired: 1 in, 3 out]
            n284 = flat-sequence {
              frame #0 {
                n285 = Wait (ms)(milliseconds to wait=10) -> ()  [unwired: 1 out]
              }
              frame #1 {
                (unwired) 6
                n286 = call "Simulate_Keyboard.vi"("Action"=2, "Virtual Key"=162) -> ()  [unwired: 7 in, 1 out]
              }
            }
          }
        }
        n287 = Divide(x=w535, y=w512) -> (x/y=w525:sgl)
        n288 = Multiply(x=w525, y=0.5) -> (x*y=w531:dbl)
        n289 = Divide(x=w534, y=w536) -> (x/y=w524:sgl)
        n290 = Multiply(x=w524, y=0.5) -> (x*y=w530:dbl)
        n291 = Unbundle(w544) -> ("X"=w526:u32, "Y"=w527:u32)
        n292 = Subtract(x=w527, y=w530) -> (x-y=w528:dbl)
        n293 = Subtract(x=w526, y=w531) -> (x-y=w529:dbl)
        n294 = Add(x=w529, y=w525) -> (x+y=w543:dbl)
        n295 = Add(x=w528, y=w524) -> (x+y=w542:dbl)
        n296 = Build Array(w469, w492, w471, w467, w463, w493, w494, w449, w448, w441, w445, w444, w447, w432, w486, w489, w499, w490, w442, w497, w485, w479, w482, w481, w477, w475, w473) -> (w495:string[])
        n297 = local write "Current \nRecord"(w495) -> ()
        n298 = event shown="[3] \"Up Button\": Mouse Down" {
          selector: _ -> [_ _ _ _ _ _ _ _ _ _ _ _ _ _ _ _]
          dyn-events: _ -> [_ _ _ _ _ _ _ _ _ _ _ _ _ _ _ _]
          timeout: 10 -> [_ _ _ _ _ _ _ _ _ _ _ _ _ _ _ _]
          tunnel: [_ _ _ _ _ _ _ _ _ _ _ _ _ TRUE _ TRUE] -> w569
          event Timeout {
            n299 = event-data() -> ()  [unwired: 1 in, 2 out]
          }
          event "Down Button": Mouse Down {
            w929 = 0
            n300 = event-data() -> ()  [unwired: 1 in, 7 out]
            n301 = local read "Data File"() -> (w945:path)
            n302 = call "Recorded Values.vi"("Path"=w945) -> ("Recorded Char"=w947:T5, "Recorded Prop"=w948:T6, "Fabrication Prop"=w946:T7)  [unwired: 8 in]
            n303 = Unbundle By Name(w947) -> ("Mobility-Sat"=w961:dbl, "Moblitity-Lin"=w962:dbl, "On/Off"=w963:dbl, "Threshold Voltage"=w964:dbl, "STS"=w965:dbl, "Trap Density-VT"=w966:dbl, "Trap Density-STS"=w967:dbl)  [unwired: 1 out]
            n304 = Unbundle By Name(w946) -> ("Date Created"=w968:string, "Material"=w949:string, "Solvent"=w950:string, "Concentration"=w951:dbl, "Method"=w952:string, "Dielectric (nm)"=w953:dbl, "Treatment"=w954:string, "Comments"=w955:string)
            n305 = Unbundle By Name(w948) -> ("Date Recorded"=w956:string, "Index"=w957:string, "Length"=w958:dbl, "Width"=w959:dbl, "Sample Temp"=w960:dbl)
            n306 = local write "Date Created"(w968) -> ()
            n307 = local write "Rec: VT-Sat"(w964) -> ()
            n308 = local write "Rec: Material"(w949) -> ()
            n309 = local write "Rec: Concentration"(w951) -> ()
            n310 = local write "Rec: Method"(w952) -> ()
            n311 = local write "Rec: Dielectric (d)"(w953) -> ()
            n312 = local write "Surface Treatment:"(w954) -> ()
            n313 = local write "Comments"(w955) -> ()
            n314 = local write "Index"(w957) -> ()
            n315 = local write "Rec: Mobility-Sat"(w961) -> ()
            n316 = local write "Rec: Mobility-Lin"(w962) -> ()
            n317 = local write "Rec: On/Off"(w963) -> ()
            n318 = local write "Rec: STS"(w965) -> ()
            n319 = local write "Rec: Trap Density-VT"(w966) -> ()
            n320 = local write "Rec: Trap Density-STS"(w967) -> ()
            n321 = local write "Rec: Solvent"(w950) -> ()
            n322 = local write "Date Recorded"(w956) -> ()
            n323 = local write "Rec: Length"(w958) -> ()
            n324 = local write "Rec: Width"(w959) -> ()
            n325 = local write "Rec: Temp"(w960) -> ()
            n326 = local read "Data File"() -> (w934:path)
            n327 = Strip Path(path=w934) -> (stripped path=w925:path, name=w943:string)
            n328 = local write "Data Folder"(w925) -> ()
            n329 = List Folder(path=w925) -> (filenames=w939:string[], error out=w879:errorcluster)  [unwired: 3 in, 2 out]
            n330 = local read "Folder Index"() -> (w881:dbl)
            n331 = property on="Image Out" class="ImageControl"() -> (error out=w882:errorcluster, "Image Center Position"=w886:cluster{"X":u32, "Y":u32})  [unwired: 2 in, 1 out]
            n332 = Array Size(array=w939) -> (size(s)=w935:i32)
            n333 = Search 1D Array(1D array=w939, element=w943) -> (index of element=w936:i32)  [unwired: 1 in]
            n334 = Decrement(x=w935) -> (x-1=w937:i32)
            n335 = Equal?(x=w936, y=w937) -> (x = y?=w938:bool)
            n336 = invoke on="Image Out" class="ImageControl" method="Clear ROI"() -> ()  [unwired: 3 in, 3 out]
            n337 = case shown="False" w938 {
              tunnel: w881 -> [w1096 _]
              tunnel: [w1095 0] -> w880
              tunnel: w879 -> [w1094 w1097]
              tunnel: [w1094 w1097] -> w878
              frame False {
                n338 = Increment(x=w1096) -> (x+1=w1095:dbl)
              }
              frame True {
              }
            }
            n339 = Unbundle(w886) -> ("X"=w884:u32)  [unwired: 1 out]
            n340 = local write "Folder Index"(w880) -> ()
            n341 = Bundle("X"=w884, 0) -> (w885:cluster{"X":u32, i32})  [unwired: 1 in]
            n342 = property on="Image Out" class="ImageControl"(error in=w882, "Image Center Position"=w885) -> ()  [unwired: 1 in, 2 out]
            n343 = Path To String(path=w925) -> (string=w944:string)
            n344 = Index Array(array=w939, index=w880) -> (element=w940:string)
            n345 = local write "Data Name:"(w940) -> ()
            n346 = Concatenate Strings(w944, "\\", w940) -> (w942:string)
            n347 = String To Path(string=w942) -> (path=w877:path)
            n348 = local read "NumPts 2"() -> (w872:dbl)
            n349 = local read "NumPts"() -> (w876:dbl)
            n350 = local write "Data File"(w877) -> ()
            n351 = call-poly <vilib>:"Read From Spreadsheet File.vi"("file path (dialog if empty)"=w877) -> ("all rows"=w931:string[][])  [unwired: 6 in, 4 out]
            n352 = call "Mobility-Vt Calculator-File.vi"("NumPts"=w876, "Path"=w877) -> ("XY Graph-Sat"=w874:cluster{dbl[], dbl[]}[], "XY Graph-Lin"=w858:cluster{dbl[], dbl[]}[], "Output"=w875:T8, "Index-Sat"=w873:dbl, "Index-Lin"=w856:dbl)  [unwired: 4 in, 1 out]
            n353 = call "STS Calculator-File.vi"("NumPts"=w872, "Path"=w877) -> ("STS Index-Sat"=w871:dbl, "XY Graph-Sat"=w870:cluster{dbl[], dbl[]}[], "Ouput"=w869:cluster{"STS-Sat":dbl, "STS-Lin":dbl})  [unwired: 5 in, 2 out]
            n354 = Unbundle By Name(w875) -> ("Mobility-Sat"=w867:dbl, "Vt-Sat"=w866:dbl, "Mobility-Lin"=w865:dbl, "Vt-Lin"=w864:dbl)
            n355 = Unbundle By Name(w869) -> ("STS-Sat"=w868:dbl)  [unwired: 1 out]
            n356 = local write "Index 2"(w871) -> ()
            n357 = local write "XY Graph 2"(w870) -> ()
            n358 = local write "MobVi Index"(w873) -> ()
            n359 = local write "Slide"(w873) -> ()
            n360 = local write "XY Graph"(w874) -> ()
            n361 = Array Size(array=w931) -> (size(s)=w930:i32[])
            n362 = local write "Calc: Mobility-Sat"(w867) -> ()
            n363 = local write "Calc: STS"(w868) -> ()
            n364 = local write "Calc: Mobility-Lin"(w864) -> ()
            n365 = local write "Calc: VT-Sat"(w866) -> ()
            n366 = local write "Calc: VT-Lin"(w865) -> ()
            n367 = Index Array(array=w930, index=w929) -> (element=w911:i32)
            n368 = Decimate 1D Array(w870) -> (w905:cluster{dbl[], dbl[]}[])  [unwired: 1 out]
            n369 = Decimate 1D Array(w874) -> (w915:cluster{dbl[], dbl[]}[])  [unwired: 1 out]
            n370 = Decimate 1D Array(w858) -> (w863:cluster{dbl[], dbl[]}[])  [unwired: 1 out]
            n371 = Array Subset(array=w931, index (row)=w929, index (col)=w929, length (col)=3) -> (w932:string[][])  [unwired: 1 in]
            n372 = Array To Cluster(array=w905) -> (cluster=w903:T9)
            n373 = Array To Cluster(array=w915) -> (cluster=w917:T9)
            n374 = Reshape Array(w932, w911) -> (w918:string[])
            n375 = Array To Cluster(array=w863) -> (cluster=w862:T9)
            n376 = Subtract(x=w911, y=20) -> (x-y=w910:i32)
            n377 = local write "New: Mobility-Sat"(w867) -> ()
            n378 = local write "New: Mobility-Lin"(w865) -> ()
            n379 = local write "New: VT-Sat"(w866) -> ()
            n380 = local write "New: VT-Lin"(w864) -> ()
            n381 = property on="Slide" class="Slide (strict)"("Scale.Maximum"=w910) -> ()  [unwired: 2 in, 2 out]
            n382 = Unbundle(w903) -> ("[0]"=w904:cluster{dbl[], dbl[]})  [unwired: 8 out]
            n383 = Unbundle(w917) -> ("[0]"=w916:cluster{dbl[], dbl[]})  [unwired: 8 out]
            n384 = Unbundle(w862) -> ("[0]"=w859:cluster{dbl[], dbl[]})  [unwired: 8 out]
            n385 = Search 1D Array(1D array=w918, element="Index:") -> (index of element=w926:i32)  [unwired: 1 in]
            n386 = local read "NumPts"() -> (w857:dbl)
            n387 = Unbundle(w859) -> (w861:dbl[], w860:dbl[])
            n388 = Increment(x=w926) -> (x+1=w927:i32)
            n389 = Unbundle(w904) -> (w902:dbl[], w901:dbl[])
            n390 = Unbundle(w916) -> (w907:dbl[], w906:dbl[])
            n391 = Array Subset(array=w861, index=w856, length=w857) -> (w855:dbl[])
            n392 = Array Subset(array=w860, index=w856, length=w857) -> (w854:dbl[])
            n393 = Array Subset(array=w902, index=w871, length=w872) -> (w909:dbl[])
            n394 = Array Subset(array=w901, index=w871, length=w872) -> (w908:dbl[])
            n395 = Array Subset(array=w907, index=w873, length=w876) -> (w914:dbl[])
            n396 = Array Subset(array=w906, index=w873, length=w876) -> (w913:dbl[])
            n397 = Index Array(array=w918, index=w927) -> (element=w890:string)
            n398 = local write "Lin-Vg Array-Used"(w855) -> ()
            n399 = local write "Sat Vg Array-Used"(w914) -> ()
            n400 = local write "Vg Array-Log-Used"(w908) -> ()
            n401 = local write "Lin Id-Used"(w854) -> ()
            n402 = local read "Image Folder"() -> (w888:path)
            n403 = local write "Sat Id-Used"(w913) -> ()
            n404 = local write "Sat Id-Log-Used"(w909) -> ()
            n405 = List Folder(path=w888, error in=w878) -> (filenames=w924:string[], error out=w891:errorcluster)  [unwired: 2 in, 2 out]
            n406 = while {
              tunnel: w924 -> [w981]
              tunnel: w890 -> [w979]
              tunnel: [w978] -> _
              tunnel: [w978] -> w923
              tunnel: w911 -> [w977]
              i -> [w978]
              stop <- w974 stop-if-true
              n407 = Index Array(array=w981, index=w978) -> (element=w982:string)
              n408 = xnode "Match Regular Expression"("input string"=w982, "regular expression"=w979) -> ("whole match"=w980:string)  [unwired: 4 in, 4 out]
              n409 = Equal?(x=w980, y=w979) -> (x = y?=w976:bool)
              n410 = Equal?(x=w977, y=w978) -> (x = y?=w975:bool)
              n411 = Or(x=w976, y=w975) -> (x .or. y?=w974:bool)
            }
            n412 = Build Path(base path=w888, name or relative path="ROI") -> (appended path=w887:path)
            n413 = Path To String(path=w888) -> (string=w921:string)
            n414 = Index Array(array=w924, index=w923) -> (element=w899:string)
            n415 = invoke on="Image Out" class="ImageControl" method="Clear ROI"(error in=w891) -> (error out=w894:errorcluster)  [unwired: 2 in, 2 out]
            n416 = local write "Image Name"(w899) -> ()
            n417 = Build Path(base path=w887, name or relative path=w890) -> (appended path=w895:path)
            n418 = call <vilib>:"Check if File or Folder Exists.vi"("error in (no error)"=w894, "path"=w895) -> ("file or folder exists?"=w892:bool, "dup path"=w893:path)  [unwired: 7 in, 1 out]
            n419 = Concatenate Strings(w921, "\\", w899) -> (w920:string)
            n420 = case shown="True" w892 {
              tunnel: w893 -> [_ w969]
              frame False {
              }
              frame True {
                n421 = Read from Text File(file (use dialog)=w969) -> (text=w973:string)  [unwired: 3 in, 3 out]
                n422 = property on="Image Out" class="ImageControl"() -> ("ROI"=w970:T10)  [unwired: 2 in, 2 out]
                n423 = Unflatten From String(type=w970, binary string=w973) -> (value=w971:T10, error out=w972:errorcluster)  [unwired: 3 in, 1 out]
                n424 = property on="Image Out" class="ImageControl"(error in=w972, "ROI"=w971) -> ()  [unwired: 1 in, 2 out]
              }
            }
            n425 = String To Path(string=w920) -> (path=w898:path)
            n426 = Empty String/Path?(string/path=w899) -> (empty?=w900:bool)
            n427 = local read "No Image"() -> (w896:path)
            n428 = Select(t=w896, s=w900, f=w898) -> (s? t:f=w897:path)
            n429 = local write "Image File"(w897) -> ()
            n430 = call "Vision Acquisition4"("Image Path"=w897) -> ("Image Out"=w922:T2)  [unwired: 25 in, 1 out]
            n431 = local write "Image Out"(w922) -> ()
            n432 = local write "Image Out 2"(w922) -> ()
          }
          event "Data File": Value Change {
            w1198 = 0
            n433 = event-data() -> ()  [unwired: 1 in, 5 out]
            n434 = local read "Data File"() -> (w1147:path)
            n435 = call "Recorded Values.vi"("Path"=w1147) -> ("Recorded Char"=w1145:T5, "Recorded Prop"=w1144:T6, "Fabrication Prop"=w1146:T7)  [unwired: 8 in]
            n436 = Unbundle By Name(w1145) -> ("Mobility-Sat"=w1131:dbl, "Moblitity-Lin"=w1130:dbl, "On/Off"=w1129:dbl, "Threshold Voltage"=w1128:dbl, "STS"=w1127:dbl, "Trap Density-VT"=w1126:dbl, "Trap Density-STS"=w1125:dbl)  [unwired: 1 out]
            n437 = Unbundle By Name(w1146) -> ("Date Created"=w1124:string, "Material"=w1143:string, "Solvent"=w1142:string, "Concentration"=w1141:dbl, "Method"=w1140:string, "Dielectric (nm)"=w1139:dbl, "Treatment"=w1138:string, "Comments"=w1137:string)
            n438 = Unbundle By Name(w1144) -> ("Date Recorded"=w1136:string, "Index"=w1135:string, "Length"=w1134:dbl, "Width"=w1133:dbl, "Sample Temp"=w1132:dbl)
            n439 = local write "Date Created"(w1124) -> ()
            n440 = local read "Data File"() -> (w1194:path)
            n441 = local write "Rec: Material"(w1143) -> ()
            n442 = local write "Rec: VT-Sat"(w1128) -> ()
            n443 = local write "Rec: Concentration"(w1141) -> ()
            n444 = local write "Rec: Method"(w1140) -> ()
            n445 = local write "Rec: Dielectric (d)"(w1139) -> ()
            n446 = local write "Surface Treatment:"(w1138) -> ()
            n447 = local write "Comments"(w1137) -> ()
            n448 = local write "Index"(w1135) -> ()
            n449 = local write "Rec: Mobility-Sat"(w1131) -> ()
            n450 = local write "Rec: Mobility-Lin"(w1130) -> ()
            n451 = local write "Rec: On/Off"(w1129) -> ()
            n452 = local write "Rec: STS"(w1127) -> ()
            n453 = local write "Rec: Trap Density-VT"(w1126) -> ()
            n454 = local write "Rec: Trap Density-STS"(w1125) -> ()
            n455 = Strip Path(path=w1194) -> (stripped path=w1193:path, name=w1207:string)
            n456 = local write "Rec: Solvent"(w1142) -> ()
            n457 = local write "Date Recorded"(w1136) -> ()
            n458 = local write "Rec: Length"(w1134) -> ()
            n459 = local write "Rec: Width"(w1133) -> ()
            n460 = local write "Rec: Temp"(w1132) -> ()
            n461 = local write "Data Folder"(w1193) -> ()
            n462 = property on="Image Out" class="ImageControl"() -> (error out=w1149:errorcluster, "Image Center Position"=w1153:cluster{"X":u32, "Y":u32})  [unwired: 2 in, 1 out]
            n463 = List Folder(path=w1193) -> (filenames=w1203:string[], error out=w1159:errorcluster)  [unwired: 3 in, 2 out]
            n464 = Search 1D Array(1D array=w1203, element=w1207) -> (index of element=w1148:i32)  [unwired: 1 in]
            n465 = local write "Folder Index"(w1148) -> ()
            n466 = Unbundle(w1153) -> ("X"=w1151:u32)  [unwired: 1 out]
            n467 = Path To String(path=w1193) -> (string=w1208:string)
            n468 = Index Array(array=w1203, index=w1148) -> (element=w1204:string)
            n469 = Bundle("X"=w1151, 0) -> (w1152:cluster{"X":u32, i32})  [unwired: 1 in]
            n470 = local write "Data Name:"(w1204) -> ()
            n471 = property on="Image Out" class="ImageControl"(error in=w1149, "Image Center Position"=w1152) -> ()  [unwired: 1 in, 2 out]
            n472 = Concatenate Strings(w1208, "\\", w1204) -> (w1206:string)
            n473 = String To Path(string=w1206) -> (path=w1123:path)
            n474 = local read "NumPts 2"() -> (w1118:dbl)
            n475 = local write "Data File"(w1123) -> ()
            n476 = local read "NumPts"() -> (w1119:dbl)
            n477 = call-poly <vilib>:"Read From Spreadsheet File.vi"("file path (dialog if empty)"=w1123) -> ("all rows"=w1200:string[][])  [unwired: 6 in, 4 out]
            n478 = call "STS Calculator-File.vi"("NumPts"=w1118, "Path"=w1123) -> ("STS Index-Sat"=w1116:dbl, "XY Graph-Sat"=w1117:cluster{dbl[], dbl[]}[], "Ouput"=w1115:cluster{"STS-Sat":dbl, "STS-Lin":dbl})  [unwired: 5 in, 2 out]
            n479 = call "Mobility-Vt Calculator-File.vi"("NumPts"=w1119, "Path"=w1123) -> ("XY Graph-Sat"=w1122:cluster{dbl[], dbl[]}[], "XY Graph-Lin"=w1111:cluster{dbl[], dbl[]}[], "Output"=w1120:T8, "Index-Sat"=w1121:dbl, "Index-Lin"=w1106:dbl)  [unwired: 4 in, 1 out]
            n480 = Unbundle By Name(w1120) -> ("Mobility-Sat"=w1102:dbl, "Vt-Sat"=w1101:dbl, "Mobility-Lin"=w1100:dbl, "Mobility-Lin"=w1099:dbl)
            n481 = local write "Index 2"(w1116) -> ()
            n482 = local write "XY Graph 2"(w1117) -> ()
            n483 = Unbundle By Name(w1115) -> ("STS-Sat"=w1114:dbl)  [unwired: 1 out]
            n484 = local write "MobVi Index"(w1121) -> ()
            n485 = Array Size(array=w1200) -> (size(s)=w1199:i32[])
            n486 = local write "Slide"(w1121) -> ()
            n487 = local write "Calc: Mobility-Sat"(w1102) -> ()
            n488 = local write "Calc: Mobility-Lin"(w1099) -> ()
            n489 = local write "Calc: VT-Sat"(w1101) -> ()
            n490 = local write "Calc: VT-Lin"(w1100) -> ()
            n491 = local write "Calc: STS"(w1114) -> ()
            n492 = Decimate 1D Array(w1111) -> (w1113:cluster{dbl[], dbl[]}[])  [unwired: 1 out]
            n493 = Decimate 1D Array(w1117) -> (w1174:cluster{dbl[], dbl[]}[])  [unwired: 1 out]
            n494 = Index Array(array=w1199, index=w1198) -> (element=w1180:i32)
            n495 = Decimate 1D Array(w1122) -> (w1183:cluster{dbl[], dbl[]}[])  [unwired: 1 out]
            n496 = local write "XY Graph"(w1122) -> ()
            n497 = Array Subset(array=w1200, index (row)=w1198, index (col)=w1198, length (col)=3) -> (w1201:string[][])  [unwired: 1 in]
            n498 = Array To Cluster(array=w1113) -> (cluster=w1112:T9)
            n499 = Array To Cluster(array=w1174) -> (cluster=w1172:T9)
            n500 = Array To Cluster(array=w1183) -> (cluster=w1185:T9)
            n501 = Reshape Array(w1201, w1180) -> (w1186:string[])
            n502 = local write "New: Mobility-Sat"(w1102) -> ()
            n503 = local write "New: Mobility-Lin"(w1100) -> ()
            n504 = Subtract(x=w1180, y=20) -> (x-y=w1178:i32)
            n505 = local write "New: VT-Sat"(w1101) -> ()
            n506 = local write "New: VT-Lin"(w1099) -> ()
            n507 = Unbundle(w1112) -> ("[0]"=w1110:cluster{dbl[], dbl[]})  [unwired: 8 out]
            n508 = property on="Slide" class="Slide (strict)"("Scale.Maximum"=w1178) -> ()  [unwired: 2 in, 2 out]
            n509 = local read "NumPts"() -> (w1107:dbl)
            n510 = Unbundle(w1110) -> (w1109:dbl[], w1108:dbl[])
            n511 = Unbundle(w1172) -> ("[0]"=w1173:cluster{dbl[], dbl[]})  [unwired: 8 out]
            n512 = Unbundle(w1185) -> ("[0]"=w1184:cluster{dbl[], dbl[]})  [unwired: 8 out]
            n513 = Search 1D Array(1D array=w1186, element="Index:") -> (index of element=w1195:i32)  [unwired: 1 in]
            n514 = local read "NumPts"() -> (w1103:dbl)
            n515 = Array Subset(array=w1109, index=w1106, length=w1107) -> (w1105:dbl[])
            n516 = Array Subset(array=w1108, index=w1106, length=w1107) -> (w1104:dbl[])
            n517 = Increment(x=w1195) -> (x+1=w1196:i32)
            n518 = Unbundle(w1173) -> (w1170:dbl[], w1169:dbl[])
            n519 = Unbundle(w1184) -> (w1171:dbl[], w1175:dbl[])
            n520 = local read "Image Folder"() -> (w1155:path)
            n521 = local write "Lin-Vg Array-Used"(w1105) -> ()
            n522 = Array Subset(array=w1170, index=w1116, length=w1118) -> (w1177:dbl[])
            n523 = Array Subset(array=w1169, index=w1116, length=w1118) -> (w1176:dbl[])
            n524 = Array Subset(array=w1171, index=w1121, length=w1103) -> (w1182:dbl[])
            n525 = Array Subset(array=w1175, index=w1121, length=w1103) -> (w1181:dbl[])
            n526 = Index Array(array=w1186, index=w1196) -> (element=w1157:string)
            n527 = local write "Lin Id-Used"(w1104) -> ()
            n528 = local write "Sat Vg Array-Used"(w1182) -> ()
            n529 = local write "Vg Array-Log-Used"(w1176) -> ()
            n530 = local write "Sat Id-Log-Used"(w1177) -> ()
            n531 = local write "Sat Id-Used"(w1181) -> ()
            n532 = local write "Index"(w1157) -> ()
            n533 = List Folder(path=w1155, error in=w1159) -> (filenames=w1191:string[], error out=w1158:errorcluster)  [unwired: 2 in, 2 out]
            n534 = Build Path(base path=w1155, name or relative path="ROI") -> (appended path=w1154:path)
            n535 = while {
              tunnel: w1191 -> [w1221]
              tunnel: w1157 -> [w1219]
              tunnel: [w1218] -> _
              tunnel: [w1218] -> w1190
              tunnel: w1180 -> [w1217]
              i -> [w1218]
              stop <- w1214 stop-if-true
              n536 = Index Array(array=w1221, index=w1218) -> (element=w1222:string)
              n537 = xnode "Match Regular Expression"("input string"=w1222, "regular expression"=w1219) -> ("whole match"=w1220:string)  [unwired: 4 in, 4 out]
              n538 = Equal?(x=w1220, y=w1219) -> (x = y?=w1216:bool)
              n539 = Equal?(x=w1217, y=w1218) -> (x = y?=w1215:bool)
              n540 = Or(x=w1216, y=w1215) -> (x .or. y?=w1214:bool)
            }
            n541 = invoke on="Image Out" class="ImageControl" method="Clear ROI"(error in=w1158) -> (error out=w1162:errorcluster)  [unwired: 2 in, 2 out]
            n542 = Build Path(base path=w1154, name or relative path=w1157) -> (appended path=w1163:path)
            n543 = call <vilib>:"Check if File or Folder Exists.vi"("error in (no error)"=w1162, "path"=w1163) -> ("file or folder exists?"=w1160:bool, "dup path"=w1161:path)  [unwired: 7 in, 1 out]
            n544 = case shown="True" w1160 {
              tunnel: w1161 -> [_ w1209]
              frame False {
              }
              frame True {
                n545 = Read from Text File(file (use dialog)=w1209) -> (text=w1213:string)  [unwired: 3 in, 3 out]
                n546 = property on="Image Out" class="ImageControl"() -> ("ROI"=w1210:T10)  [unwired: 2 in, 2 out]
                n547 = Unflatten From String(type=w1210, binary string=w1213) -> (value=w1211:T10, error out=w1212:errorcluster)  [unwired: 3 in, 1 out]
                n548 = property on="Image Out" class="ImageControl"(error in=w1212, "ROI"=w1211) -> ()  [unwired: 1 in, 2 out]
              }
            }
            n549 = invoke on="Image Out" class="ImageControl" method="Clear ROI"() -> ()  [unwired: 3 in, 3 out]
            n550 = Path To String(path=w1155) -> (string=w1189:string)
            n551 = Index Array(array=w1191, index=w1190) -> (element=w1167:string)
            n552 = Concatenate Strings(w1189, "\\", w1167) -> (w1188:string)
            n553 = local write "Image Name"(w1167) -> ()
            n554 = String To Path(string=w1188) -> (path=w1166:path)
            n555 = Empty String/Path?(string/path=w1167) -> (empty?=w1168:bool)
            n556 = local read "No Image"() -> (w1164:path)
            n557 = Select(t=w1164, s=w1168, f=w1166) -> (s? t:f=w1165:path)
            n558 = local write "Image File"(w1165) -> ()
            n559 = call "Vision Acquisition3"("Image Path"=w1165) -> ("Image Out"=w1192:T2)  [unwired: 25 in, 1 out]
            n560 = local write "Image Out"(w1192) -> ()
            n561 = local write "Image Out 2"(w1192) -> ()
          }
          event "Up Button": Mouse Down {
            w1434 = 0
            n562 = event-data() -> ()  [unwired: 1 in, 5 out]
            n563 = local read "Data File"() -> (w1381:path)
            n564 = call "Recorded Values.vi"("Path"=w1381) -> ("Recorded Char"=w1379:T5, "Recorded Prop"=w1378:T6, "Fabrication Prop"=w1380:T7)  [unwired: 8 in]
            n565 = Unbundle By Name(w1379) -> ("Mobility-Sat"=w1365:dbl, "Moblitity-Lin"=w1364:dbl, "On/Off"=w1363:dbl, "Threshold Voltage"=w1362:dbl, "STS"=w1361:dbl, "Trap Density-VT"=w1360:dbl, "Trap Density-STS"=w1359:dbl)  [unwired: 1 out]
            n566 = Unbundle By Name(w1380) -> ("Date Created"=w1358:string, "Material"=w1377:string, "Solvent"=w1376:string, "Concentration"=w1375:dbl, "Method"=w1374:string, "Dielectric (nm)"=w1373:dbl, "Treatment"=w1372:string, "Comments"=w1371:string)
            n567 = Unbundle By Name(w1378) -> ("Date Recorded"=w1370:string, "Index"=w1369:string, "Length"=w1368:dbl, "Width"=w1367:dbl, "Sample Temp"=w1366:dbl)
            n568 = local write "Date Created"(w1358) -> ()
            n569 = local write "Rec: Material"(w1377) -> ()
            n570 = local write "Rec: VT-Sat"(w1362) -> ()
            n571 = local write "Rec: Solvent"(w1376) -> ()
            n572 = local write "Rec: Concentration"(w1375) -> ()
            n573 = local write "Rec: Method"(w1374) -> ()
            n574 = local write "Rec: Dielectric (d)"(w1373) -> ()
            n575 = local write "Surface Treatment:"(w1372) -> ()
            n576 = local write "Comments"(w1371) -> ()
            n577 = local write "Index"(w1369) -> ()
            n578 = local write "Rec: Mobility-Sat"(w1365) -> ()
            n579 = local write "Rec: Mobility-Lin"(w1364) -> ()
            n580 = local write "Rec: On/Off"(w1363) -> ()
            n581 = local write "Rec: STS"(w1361) -> ()
            n582 = local write "Rec: Trap Density-VT"(w1360) -> ()
            n583 = local write "Rec: Trap Density-STS"(w1359) -> ()
            n584 = local write "Date Recorded"(w1370) -> ()
            n585 = local write "Rec: Length"(w1368) -> ()
            n586 = local write "Rec: Width"(w1367) -> ()
            n587 = local write "Rec: Temp"(w1366) -> ()
            n588 = local read "Data File"() -> (w1430:path)
            n589 = Strip Path(path=w1430) -> (stripped path=w1429:path, name=w1445:string)
            n590 = local write "Data Folder"(w1429) -> ()
            n591 = List Folder(path=w1429) -> (filenames=w1439:string[], error out=w1396:errorcluster)  [unwired: 3 in, 2 out]
            n592 = Array Size(array=w1439) -> (size(s)=w1384:i32)
            n593 = Search 1D Array(1D array=w1439, element=w1445) -> (index of element=w1440:i32)  [unwired: 1 in]
            n594 = Equal To 0?(x=w1440) -> (x = 0?=w1441:bool)
            n595 = local read "Folder Index"() -> (w1383:dbl)
            n596 = property on="Image Out" class="ImageControl"() -> (error out=w1386:errorcluster, "Image Center Position"=w1390:cluster{"X":u32, "Y":u32})  [unwired: 2 in, 1 out]
            n597 = case shown="True" w1441 {
              tunnel: w1383 -> [w1573 _]
              tunnel: [w1572 w1574] -> w1382
              tunnel: w1384 -> [_ w1575]
              frame False {
                n598 = Decrement(x=w1573) -> (x-1=w1572:dbl)
              }
              frame True {
                n599 = Decrement(x=w1575) -> (x-1=w1574:i32)
              }
            }
            n600 = local write "Folder Index"(w1382) -> ()
            n601 = Unbundle(w1390) -> ("X"=w1388:u32)  [unwired: 1 out]
            n602 = Bundle("X"=w1388, 0) -> (w1389:cluster{"X":u32, i32})  [unwired: 1 in]
            n603 = Path To String(path=w1429) -> (string=w1446:string)
            n604 = Index Array(array=w1439, index=w1382) -> (element=w1442:string)
            n605 = local write "Data Name:"(w1442) -> ()
            n606 = property on="Image Out" class="ImageControl"(error in=w1386, "Image Center Position"=w1389) -> ()  [unwired: 1 in, 2 out]
            n607 = Concatenate Strings(w1446, "\\", w1442) -> (w1444:string)
            n608 = String To Path(string=w1444) -> (path=w1357:path)
            n609 = local read "NumPts 2"() -> (w1352:dbl)
            n610 = local write "Data File"(w1357) -> ()
            n611 = local read "NumPts"() -> (w1356:dbl)
            n612 = call "Mobility-Vt Calculator-File.vi"("NumPts"=w1356, "Path"=w1357) -> ("XY Graph-Sat"=w1354:cluster{dbl[], dbl[]}[], "XY Graph-Lin"=w1338:cluster{dbl[], dbl[]}[], "Output"=w1355:T8, "Index-Sat"=w1353:dbl, "Index-Lin"=w1339:dbl)  [unwired: 4 in, 1 out]
            n613 = call "STS Calculator-File.vi"("NumPts"=w1352, "Path"=w1357) -> ("STS Index-Sat"=w1351:dbl, "XY Graph-Sat"=w1350:cluster{dbl[], dbl[]}[], "Ouput"=w1349:cluster{"STS-Sat":dbl, "STS-Lin":dbl})  [unwired: 5 in, 2 out]
            n614 = call-poly <vilib>:"Read From Spreadsheet File.vi"("file path (dialog if empty)"=w1357) -> ("all rows"=w1436:string[][])  [unwired: 6 in, 4 out]
            n615 = Unbundle By Name(w1355) -> ("Mobility-Sat"=w1337:dbl, "Vt-Sat"=w1336:dbl, "Mobility-Lin"=w1335:dbl, "Mobility-Lin"=w1334:dbl)
            n616 = Unbundle By Name(w1349) -> ("STS-Sat"=w1348:dbl)  [unwired: 1 out]
            n617 = local write "Index 2"(w1351) -> ()
            n618 = local write "XY Graph 2"(w1350) -> ()
            n619 = local write "MobVi Index"(w1353) -> ()
            n620 = local write "Slide"(w1353) -> ()
            n621 = local write "XY Graph"(w1354) -> ()
            n622 = Array Size(array=w1436) -> (size(s)=w1435:i32[])
            n623 = local write "Calc: Mobility-Sat"(w1337) -> ()
            n624 = local write "Calc: Mobility-Lin"(w1334) -> ()
            n625 = local write "Calc: VT-Sat"(w1336) -> ()
            n626 = local write "Calc: VT-Lin"(w1335) -> ()
            n627 = local write "Calc: STS"(w1348) -> ()
            n628 = Decimate 1D Array(w1338) -> (w1347:cluster{dbl[], dbl[]}[])  [unwired: 1 out]
            n629 = Decimate 1D Array(w1350) -> (w1413:cluster{dbl[], dbl[]}[])  [unwired: 1 out]
            n630 = Index Array(array=w1435, index=w1434) -> (element=w1419:i32)
            n631 = Decimate 1D Array(w1354) -> (w1423:cluster{dbl[], dbl[]}[])  [unwired: 1 out]
            n632 = Array To Cluster(array=w1347) -> (cluster=w1346:T9)
            n633 = Array Subset(array=w1436, index (row)=w1434, index (col)=w1434, length (col)=3) -> (w1437:string[][])  [unwired: 1 in]
            n634 = local write "New: Mobility-Sat"(w1337) -> ()
            n635 = local write "New: Mobility-Lin"(w1335) -> ()
            n636 = Array To Cluster(array=w1413) -> (cluster=w1411:T9)
            n637 = Array To Cluster(array=w1423) -> (cluster=w1425:T9)
            n638 = Reshape Array(w1437, w1419) -> (w1426:string[])
            n639 = local write "New: VT-Sat"(w1336) -> ()
            n640 = local write "New: VT-Lin"(w1334) -> ()
            n641 = Subtract(x=w1419, y=20) -> (x-y=w1418:i32)
            n642 = Unbundle(w1346) -> ("[0]"=w1343:cluster{dbl[], dbl[]})  [unwired: 8 out]
            n643 = property on="Slide" class="Slide (strict)"("Scale.Maximum"=w1418) -> ()  [unwired: 2 in, 2 out]
            n644 = Unbundle(w1411) -> ("[0]"=w1412:cluster{dbl[], dbl[]})  [unwired: 8 out]
            n645 = Unbundle(w1425) -> ("[0]"=w1424:cluster{dbl[], dbl[]})  [unwired: 8 out]
            n646 = local read "NumPts"() -> (w1340:dbl)
            n647 = Unbundle(w1343) -> (w1342:dbl[], w1341:dbl[])
            n648 = Search 1D Array(1D array=w1426, element="Index:") -> (index of element=w1431:i32)  [unwired: 1 in]
            n649 = Increment(x=w1431) -> (x+1=w1432:i32)
            n650 = Unbundle(w1412) -> (w1410:dbl[], w1409:dbl[])
            n651 = Unbundle(w1424) -> (w1417:dbl[], w1416:dbl[])
            n652 = Array Subset(array=w1342, index=w1339, length=w1340) -> (w1344:dbl[])
            n653 = Array Subset(array=w1341, index=w1339, length=w1340) -> (w1345:dbl[])
            n654 = local read "Image Folder"() -> (w1385:path)
            n655 = local write "Lin-Vg Array-Used"(w1344) -> ()
            n656 = Array Subset(array=w1410, index=w1351, length=w1352) -> (w1415:dbl[])
            n657 = Array Subset(array=w1409, index=w1351, length=w1352) -> (w1414:dbl[])
            n658 = Array Subset(array=w1417, index=w1353, length=w1356) -> (w1422:dbl[])
            n659 = Array Subset(array=w1416, index=w1353, length=w1356) -> (w1421:dbl[])
            n660 = local write "Lin Id-Used"(w1345) -> ()
            n661 = Index Array(array=w1426, index=w1432) -> (element=w1392:string)
            n662 = local write "Sat Vg Array-Used"(w1422) -> ()
            n663 = local write "Vg Array-Log-Used"(w1414) -> ()
            n664 = local write "Sat Id-Log-Used"(w1415) -> ()
            n665 = local write "Sat Id-Used"(w1421) -> ()
            n666 = local write "Index"(w1392) -> ()
            n667 = List Folder(path=w1385, error in=w1396) -> (filenames=w1428:string[], error out=w1395:errorcluster)  [unwired: 2 in, 2 out]
            n668 = Build Path(base path=w1385, name or relative path="ROI") -> (appended path=w1393:path)
            n669 = while {
              tunnel: w1428 -> [w1459]
              tunnel: w1392 -> [w1457]
              tunnel: [w1456] -> w1427
              tunnel: w1419 -> [w1455]
              i -> [w1456]
              stop <- w1452 stop-if-true
              n670 = Index Array(array=w1459, index=w1456) -> (element=w1460:string)
              n671 = xnode "Match Regular Expression"("input string"=w1460, "regular expression"=w1457) -> ("whole match"=w1458:string)  [unwired: 4 in, 4 out]
              n672 = Equal?(x=w1458, y=w1457) -> (x = y?=w1454:bool)
              n673 = Equal?(x=w1455, y=w1456) -> (x = y?=w1453:bool)
              n674 = Or(x=w1454, y=w1453) -> (x .or. y?=w1452:bool)
            }
            n675 = invoke on="Image Out" class="ImageControl" method="Clear ROI"(error in=w1395) -> (error out=w1399:errorcluster)  [unwired: 2 in, 2 out]
            n676 = Build Path(base path=w1393, name or relative path=w1392) -> (appended path=w1391:path)
            n677 = call <vilib>:"Check if File or Folder Exists.vi"("error in (no error)"=w1399, "path"=w1391) -> ("file or folder exists?"=w1397:bool, "dup path"=w1398:path)  [unwired: 7 in, 1 out]
            n678 = case shown="True" w1397 {
              tunnel: w1398 -> [_ w1447]
              frame False {
              }
              frame True {
                n679 = Read from Text File(file (use dialog)=w1447) -> (text=w1451:string)  [unwired: 3 in, 3 out]
                n680 = property on="Image Out" class="ImageControl"() -> ("ROI"=w1448:T10)  [unwired: 2 in, 2 out]
                n681 = Unflatten From String(type=w1448, binary string=w1451) -> (value=w1449:T10, error out=w1450:errorcluster)  [unwired: 3 in, 1 out]
                n682 = property on="Image Out" class="ImageControl"(error in=w1450, "ROI"=w1449) -> ()  [unwired: 1 in, 2 out]
              }
            }
            n683 = Index Array(array=w1428, index=w1427) -> (element=w1401:string)
            n684 = local write "Image Name"(w1401) -> ()
            n685 = Empty String/Path?(string/path=w1401) -> (empty?=w1408:bool)
            n686 = Build Path(base path=w1385, name or relative path=w1401) -> (appended path=w1400:path)
            n687 = local read "No Image"() -> (w1407:path)
            n688 = Select(t=w1407, s=w1408, f=w1400) -> (s? t:f=w1402:path)
            n689 = call <vilib>:"Get File Extension.vi"("file"=w1402) -> ("lowercase file extension"=w1404:string)  [unwired: 7 in, 3 out]
            n690 = local write "Image File"(w1402) -> ()
            n691 = local write "String"(w1404) -> ()
            n692 = Search 1D Array(1D array=string[] ["bmp", "jpeg", "png", "jpg", "gif"], element=w1404) -> (index of element=w1403:i32)  [unwired: 1 in]
            n693 = call "Vision Acquisition5"("Image Path"=w1402) -> ("Image Out"=w1406:T2)  [unwired: 25 in, 1 out]
            n694 = Less Than 0?(x=w1403) -> ()  [unwired: 1 out]
            n695 = local write "Image Out"(w1406) -> ()
            n696 = local write "Image Out 2"(w1406) -> ()
          }
          event "Save Changes? 3": Mouse Down {
            n697 = event-data() -> ()  [unwired: 1 in, 7 out]
            n698 = local read "Image Folder"() -> (w1576:path)
            n699 = Build Path(base path=w1576, name or relative path="ROI") -> (appended path=w1583:path)
            n700 = call <vilib>:"Check if File or Folder Exists.vi"("path"=w1583) -> ("file or folder exists?"=w1585:bool, "dup path"=w1582:path)  [unwired: 8 in, 1 out]
            n701 = case shown="False" w1585 {
              tunnel: w1582 -> [w1587 w1588]
              tunnel: [w1586 w1588] -> w1577
              frame False {
                n702 = Create Folder(path (use dialog)=w1587) -> (created path=w1586:path)  [unwired: 2 in, 2 out]
              }
              frame True {
              }
            }
            n703 = local read "Index"() -> (w1579:string)
            n704 = property on="Image Out" class="ImageControl"() -> ("ROI"=w1581:T10)  [unwired: 2 in, 2 out]
            n705 = Build Path(base path=w1577, name or relative path=w1579) -> (appended path=w1578:path)
            n706 = Flatten To String(anything=w1581) -> (data string=w1580:string)  [unwired: 3 in, 2 out]
            n707 = Write to Text File(file (use dialog)=w1578, text=w1580) -> ()  [unwired: 2 in, 3 out]
          }
          event "Next Button": Mouse Down {
            n708 = event-data() -> ()  [unwired: 1 in, 5 out]
            n709 = local read "XY Graph"() -> (w1601:cluster{dbl[], dbl[]}[])
            n710 = Decimate 1D Array(w1601) -> (w1597:cluster{dbl[], dbl[]}[], w1596:cluster{dbl[], dbl[]}[])
            n711 = Array To Cluster(array=w1597) -> (cluster=w1607:T9)
            n712 = local read "MobVi Index"() -> (w1603:dbl)
            n713 = Unbundle(w1607) -> ("[0]"=w1606:cluster{dbl[], dbl[]})  [unwired: 8 out]
            n714 = local read "NumPts"() -> (w1602:dbl)
            n715 = Unbundle(w1606) -> (w1605:dbl[], w1604:dbl[])
            n716 = Increment(x=w1603) -> (x+1=w1598:dbl)
            n717 = local read "New: Dielectric"() -> (w1592:dbl)
            n718 = local read "New: Length"() -> (w1591:dbl)
            n719 = local read "New: Width"() -> (w1590:dbl)
            n720 = local write "MobVi Index"(w1598) -> ()
            n721 = Array Subset(array=w1605, index=w1598, length=w1602) -> (w1594:dbl[])
            n722 = Array Subset(array=w1604, index=w1598, length=w1602) -> (w1593:dbl[])
            n723 = local write "Sat Vg Array-Used"(w1594) -> ()
            n724 = local write "Sat Id-Used"(w1593) -> ()
            n725 = call "Mobility-Vt-Used Pts_Linear.vi"("Width"=w1590, "Length"=w1591, "Dielectric (d)"=w1592, "Sat Id Used"=w1593, "Vg Used"=w1594) -> ("Vt"=w1589:dbl, "Mobility"=w1595:dbl)  [unwired: 4 in, 1 out]
            n726 = Bundle(w1594, w1593) -> (w1600:cluster{dbl[], dbl[]})  [unwired: 1 in]
            n727 = local write "New: VT-Sat"(w1589) -> ()
            n728 = local write "New: Mobility-Sat"(w1595) -> ()
            n729 = Build Array (concatenate)(w1597, w1596, w1600) -> (w1599:cluster{dbl[], dbl[]}[])
            n730 = local write "XY Graph"(w1599) -> ()
          }
          event "Next Button 2": Mouse Down {
            n731 = event-data() -> ()  [unwired: 1 in, 7 out]
            n732 = local read "XY Graph 2"() -> (w1616:cluster{dbl[], dbl[]}[])
            n733 = Decimate 1D Array(w1616) -> (w1612:cluster{dbl[], dbl[]}[], w1611:cluster{dbl[], dbl[]}[])
            n734 = Array To Cluster(array=w1612) -> (cluster=w1622:T9)
            n735 = local read "Index 2"() -> (w1618:dbl)
            n736 = Unbundle(w1622) -> ("[0]"=w1621:cluster{dbl[], dbl[]})  [unwired: 8 out]
            n737 = local read "NumPts 2"() -> (w1617:dbl)
            n738 = Unbundle(w1621) -> (w1620:dbl[], w1619:dbl[])
            n739 = Increment(x=w1618) -> (x+1=w1613:dbl)
            n740 = local write "Index 2"(w1613) -> ()
            n741 = Array Subset(array=w1620, index=w1613, length=w1617) -> (w1609:dbl[])
            n742 = Array Subset(array=w1619, index=w1613, length=w1617) -> (w1608:dbl[])
            n743 = local write "Vg Array-Log-Used"(w1608) -> ()
            n744 = local write "Sat Id-Log-Used"(w1609) -> ()
            n745 = Bundle(w1609, w1608) -> (w1615:cluster{dbl[], dbl[]})  [unwired: 1 in]
            n746 = call "STS-Used.vi"("Id Used"=w1609, "Vg-Used"=w1608) -> ("STS"=w1610:dbl)  [unwired: 9 in]
            n747 = Build Array (concatenate)(w1612, w1611, w1615) -> (w1614:cluster{dbl[], dbl[]}[])
            n748 = local write "New: STS"(w1610) -> ()
            n749 = local write "XY Graph 2"(w1614) -> ()
          }
          event "Previous Button 2": Mouse Down {
            n750 = event-data() -> ()  [unwired: 1 in, 7 out]
            n751 = local read "XY Graph 2"() -> (w1632:cluster{dbl[], dbl[]}[])
            n752 = Decimate 1D Array(w1632) -> (w1629:cluster{dbl[], dbl[]}[], w1628:cluster{dbl[], dbl[]}[])
            n753 = Array To Cluster(array=w1629) -> (cluster=w1637:T9)
            n754 = local read "Index 2"() -> (w1625:dbl)
            n755 = Unbundle(w1637) -> ("[0]"=w1636:cluster{dbl[], dbl[]})  [unwired: 8 out]
            n756 = local read "NumPts 2"() -> (w1633:dbl)
            n757 = Unbundle(w1636) -> (w1635:dbl[], w1634:dbl[])
            n758 = Decrement(x=w1625) -> (x-1=w1626:dbl)
            n759 = local write "Index 2"(w1626) -> ()
            n760 = Array Subset(array=w1635, index=w1626, length=w1633) -> (w1623:dbl[])
            n761 = Array Subset(array=w1634, index=w1626, length=w1633) -> (w1624:dbl[])
            n762 = local write "Vg Array-Log-Used"(w1624) -> ()
            n763 = local write "Sat Id-Log-Used"(w1623) -> ()
            n764 = Bundle(w1623, w1624) -> (w1631:cluster{dbl[], dbl[]})  [unwired: 1 in]
            n765 = call "STS-Used.vi"("Id Used"=w1623, "Vg-Used"=w1624) -> ("STS"=w1627:dbl)  [unwired: 9 in]
            n766 = Build Array (concatenate)(w1629, w1628, w1631) -> (w1630:cluster{dbl[], dbl[]}[])
            n767 = local write "New: STS"(w1627) -> ()
            n768 = local write "XY Graph 2"(w1630) -> ()
          }
          event "Previous Button": Mouse Down {
            n769 = event-data() -> ()  [unwired: 1 in, 5 out]
            n770 = local read "XY Graph"() -> (w1651:cluster{dbl[], dbl[]}[])
            n771 = Decimate 1D Array(w1651) -> (w1648:cluster{dbl[], dbl[]}[], w1647:cluster{dbl[], dbl[]}[])
            n772 = Array To Cluster(array=w1648) -> (cluster=w1656:T9)
            n773 = local read "MobVi Index"() -> (w1646:dbl)
            n774 = Unbundle(w1656) -> ("[0]"=w1655:cluster{dbl[], dbl[]})  [unwired: 8 out]
            n775 = local read "NumPts"() -> (w1652:dbl)
            n776 = Unbundle(w1655) -> (w1654:dbl[], w1653:dbl[])
            n777 = Decrement(x=w1646) -> (x-1=w1645:dbl)
            n778 = local read "New: Dielectric"() -> (w1639:dbl)
            n779 = local read "New: Length"() -> (w1640:dbl)
            n780 = local read "New: Width"() -> (w1641:dbl)
            n781 = local write "MobVi Index"(w1645) -> ()
            n782 = Array Subset(array=w1654, index=w1645, length=w1652) -> (w1644:dbl[])
            n783 = Array Subset(array=w1653, index=w1645, length=w1652) -> (w1643:dbl[])
            n784 = local write "Sat Vg Array-Used"(w1644) -> ()
            n785 = local write "Sat Id-Used"(w1643) -> ()
            n786 = call "Mobility-Vt-Used Pts_Linear.vi"("Width"=w1641, "Length"=w1640, "Dielectric (d)"=w1639, "Sat Id Used"=w1643, "Vg Used"=w1644) -> ("Vt"=w1638:dbl, "Mobility"=w1642:dbl)  [unwired: 4 in, 1 out]
            n787 = Bundle(w1644, w1643) -> (w1650:cluster{dbl[], dbl[]})  [unwired: 1 in]
            n788 = local write "New: VT-Sat"(w1638) -> ()
            n789 = Build Array (concatenate)(w1648, w1647, w1650) -> (w1649:cluster{dbl[], dbl[]}[])
            n790 = local write "New: Mobility-Sat"(w1642) -> ()
            n791 = local write "XY Graph"(w1649) -> ()
          }
          event "Slide": Value Change {
            n792 = event-data() -> ()  [unwired: 1 in, 5 out]
            n793 = local read "XY Graph"() -> (w1669:cluster{dbl[], dbl[]}[])
            n794 = Decimate 1D Array(w1669) -> (w1666:cluster{dbl[], dbl[]}[], w1665:cluster{dbl[], dbl[]}[])
            n795 = Array To Cluster(array=w1666) -> (cluster=w1674:T9)
            n796 = Unbundle(w1674) -> ("[0]"=w1673:cluster{dbl[], dbl[]})  [unwired: 8 out]
            n797 = local read "NumPts"() -> (w1670:dbl)
            n798 = local read "Slide"() -> (w1658:dbl)
            n799 = Unbundle(w1673) -> (w1672:dbl[], w1671:dbl[])
            n800 = local read "New: Dielectric"() -> (w1659:dbl)
            n801 = local read "New: Length"() -> (w1660:dbl)
            n802 = local read "New: Width"() -> (w1661:dbl)
            n803 = local write "MobVi Index"(w1658) -> ()
            n804 = Array Subset(array=w1672, index=w1658, length=w1670) -> (w1664:dbl[])
            n805 = Array Subset(array=w1671, index=w1658, length=w1670) -> (w1663:dbl[])
            n806 = local write "Sat Vg Array-Used"(w1664) -> ()
            n807 = local write "Sat Id-Used"(w1663) -> ()
            n808 = call "Mobility-Vt-Used Pts_Linear.vi"("Width"=w1661, "Length"=w1660, "Dielectric (d)"=w1659, "Sat Id Used"=w1663, "Vg Used"=w1664) -> ("Vt"=w1657:dbl, "Mobility"=w1662:dbl)  [unwired: 4 in, 1 out]
            n809 = Bundle(w1664, w1663) -> (w1668:cluster{dbl[], dbl[]})  [unwired: 1 in]
            n810 = local write "New: VT-Sat"(w1657) -> ()
            n811 = Build Array (concatenate)(w1666, w1665, w1668) -> (w1667:cluster{dbl[], dbl[]}[])
            n812 = local write "New: Mobility-Sat"(w1662) -> ()
            n813 = local write "XY Graph"(w1667) -> ()
          }
          event "Slide 2": Value Change {
            n814 = event-data() -> ()  [unwired: 1 in, 5 out]
            n815 = local read "XY Graph 2"() -> (w1683:cluster{dbl[], dbl[]}[])
            n816 = Decimate 1D Array(w1683) -> (w1680:cluster{dbl[], dbl[]}[], w1679:cluster{dbl[], dbl[]}[])
            n817 = Array To Cluster(array=w1680) -> (cluster=w1688:T9)
            n818 = Unbundle(w1688) -> ("[0]"=w1687:cluster{dbl[], dbl[]})  [unwired: 8 out]
            n819 = local read "NumPts 2"() -> (w1684:dbl)
            n820 = local read "Slide 2"() -> (w1678:dbl)
            n821 = Unbundle(w1687) -> (w1686:dbl[], w1685:dbl[])
            n822 = local write "Index 2"(w1678) -> ()
            n823 = Array Subset(array=w1686, index=w1678, length=w1684) -> (w1676:dbl[])
            n824 = Array Subset(array=w1685, index=w1678, length=w1684) -> (w1675:dbl[])
            n825 = local write "Vg Array-Log-Used"(w1675) -> ()
            n826 = local write "Sat Id-Log-Used"(w1676) -> ()
            n827 = call "STS-Used.vi"("Id Used"=w1676, "Vg-Used"=w1675) -> ("STS"=w1677:dbl)  [unwired: 9 in]
            n828 = Bundle(w1676, w1675) -> (w1682:cluster{dbl[], dbl[]})  [unwired: 1 in]
            n829 = local write "New: STS"(w1677) -> ()
            n830 = Build Array (concatenate)(w1680, w1679, w1682) -> (w1681:cluster{dbl[], dbl[]}[])
            n831 = local write "XY Graph 2"(w1681) -> ()
          }
          event "Save Changes?": Mouse Down {
            n832 = event-data() -> ()  [unwired: 1 in, 5 out]
            n833 = flat-sequence {
              tunnel: [w1719] -> w1694
              tunnel: [w1718] -> w1692
              tunnel: [w1718] -> w1691
              tunnel: [w1701] -> w1689
              tunnel: w1694 -> [w1833]
              tunnel: [w1834] -> w1693
              tunnel: w1692 -> [w1834]
              tunnel: w1691 -> [w1832]
              tunnel: [w1830] -> w1690
              tunnel: w1689 -> [w1830]
              tunnel: w1693 -> [w1839]
              tunnel: w1690 -> [w1838]
              frame #0 {
                w1706 = -1
                w1699 = "S.T.S. (V/decade):"
                w1700 = "Threshold V (V):"
                (unwired) 3
                w1704 = 1
                n834 = local read "Rec: Temp"() -> (w1697:dbl)
                n835 = Equal To 0?(x=w1697) -> (x = 0?=w1696:bool)
                n836 = case shown="False" w1696 {
                  tunnel: [w1745 ""] -> w1695
                  frame False {
                    n837 = local read "Rec: Temp"() -> (w1747:dbl)
                    n838 = Number To Decimal String(number=w1747) -> (decimal integer string=w1744:string)  [unwired: 1 in]
                    n839 = Concatenate Strings("_", w1744, "K") -> (w1745:string)
                  }
                  frame True {
                  }
                }
                n840 = flat-sequence {
                  tunnel: [w1761] -> w1698
                  tunnel: w1698 -> [w1778]
                  frame #0 {
                    # "Makes Empty File for Transformer Data"
                    n841 = local read "Data Folder"() -> (w1750:path)
                    n842 = Build Path(base path=w1750, name or relative path="Stats") -> (appended path=w1752:path)
                    n843 = call <vilib>:"Check if File or Folder Exists.vi"("path"=w1752) -> ("file or folder exists?"=w1753:bool, "dup path"=w1754:path)  [unwired: 8 in, 1 out]
                    n844 = case shown="False" w1753 {
                      tunnel: [w1758 w1760] -> w1755
                      tunnel: w1754 -> [w1759 w1760]
                      frame False {
                        n845 = Create Folder(path (use dialog)=w1759) -> (created path=w1758:path)  [unwired: 2 in, 2 out]
                      }
                      frame True {
                      }
                    }
                    n846 = Build Path(base path=w1755, name or relative path="Tranformer Data.txt") -> (appended path=w1757:path)
                    n847 = call-poly <vilib>:"Write To Spreadsheet File.vi"("append to file? (new file:F)"=TRUE, "file path (dialog if empty)"=w1757) -> ()  [unwired: 6 in, 1 out]
                  }
                  frame #1 {
                    # "Adds Headers if they don't exist"
                    n848 = Concatenate Strings("Stats\\", "Tranformer Data.txt") -> (w1768:string)
                    n849 = local read "Data Folder"() -> (w1767:path)
                    n850 = Build Path(base path=w1767, name or relative path=w1768) -> (appended path=w1761:path)
                    n851 = call-poly <vilib>:"Read From Spreadsheet File.vi"("file path (dialog if empty)"=w1761) -> ("first row"=w1766:string[])  [unwired: 6 in, 4 out]
                    n852 = Search 1D Array(1D array=w1766, element="DeviceID") -> (index of element=w1764:i32)  [unwired: 1 in]
                    n853 = Equal?(x=w1764, y=0) -> (x = y?=w1762:bool)
                    n854 = case shown="False" w1762 {
                      tunnel: w1761 -> [w1772 _]
                      frame False {
                        n855 = local read "Transformer \nHeaders"() -> (w1771:string[])
                        n856 = call-poly <vilib>:"Write To Spreadsheet File.vi"("1D data"=w1771, "file path (dialog if empty)"=w1772) -> ()  [unwired: 6 in, 1 out]
                      }
                      frame True {
                      }
                    }
                  }
                  frame #2 {
                    # "Adds current device if it doesn't exist"
                    n857 = local read "Current \nRecord"() -> (w1777:string[])
                    n858 = Index Array(array=w1777, index=0) -> (element=w1776:string)
                    n859 = Concatenate Strings("Stats\\", "Tranformer Data.txt") -> (w1781:string)
                    n860 = local read "Data Folder"() -> (w1780:path)
                    n861 = local write "Current Device ID"(w1776) -> ()
                    n862 = local read "Current Device ID"() -> (w1786:string)
                    n863 = Build Path(base path=w1780, name or relative path=w1781) -> (appended path=w1779:path)
                    n864 = call-poly <vilib>:"Read From Spreadsheet File.vi"("file path (dialog if empty)"=w1779) -> ("all rows"=w1773:string[][])  [unwired: 6 in, 4 out]
                    n865 = Index Array(array=w1773, index (col)=0) -> (element=w1774:string[])  [unwired: 1 in]
                    n866 = Search 1D Array(1D array=w1774, element=w1786) -> (index of element=w1775:i32)  [unwired: 1 in]
                    n867 = Equal?(x=w1775, y=-1) -> (x = y?=w1788:bool)
                    n868 = case shown="False" w1788 {
                      tunnel: w1778 -> [w1791 w1802]
                      tunnel: w1775 -> [w1794 _]
                      tunnel: w1773 -> [w1795 _]
                      frame False {
                        n869 = local read "Current \nRecord"() -> (w1793:string[])
                        n870 = Replace Array Subset(array=w1795, new element=w1793, index (row)=w1794) -> (w1792:string[][])  [unwired: 1 in]
                        n871 = flat-sequence {
                          tunnel: w1791 -> [w1796]
                          tunnel: w1792 -> [w1797]
                          tunnel: [w1797] -> w1790
                          tunnel: [w1796] -> w1789
                          tunnel: w1790 -> [w1799]
                          tunnel: w1789 -> [w1798]
                          frame #0 {
                            n872 = Delete(path (use dialog)=w1796) -> ()  [unwired: 4 in, 3 out]
                          }
                          frame #1 {
                            n873 = call-poly <vilib>:"Write To Spreadsheet File.vi"("append to file? (new file:F)"=TRUE, "2D data"=w1799, "file path (dialog if empty)"=w1798) -> ()  [unwired: 5 in, 1 out]
                          }
                        }
                      }
                      frame True {
                        n874 = local read "Current \nRecord"() -> (w1801:string[])
                        n875 = call-poly <vilib>:"Write To Spreadsheet File.vi"("append to file? (new file:F)"=TRUE, "1D data"=w1801, "file path (dialog if empty)"=w1802) -> ()  [unwired: 5 in, 1 out]
                      }
                    }
                  }
                }
                n876 = local read "New: Length"() -> (w1730:dbl)
                n877 = local read "Data File"() -> (w1719:path)
                n878 = call-poly <vilib>:"Read From Spreadsheet File.vi"("file path (dialog if empty)"=w1719) -> ("all rows"=w1711:string[][])  [unwired: 6 in, 4 out]
                n879 = Number To Fractional String(number=w1730) -> (F-format string=w1722:string)  [unwired: 3 in]
                n880 = local read "New: Width"() -> (w1732:dbl)
                n881 = Array Size(array=w1711) -> (size(s)=w1713:i32[])
                n882 = local read "New: Mobility-Sat"() -> (w1741:dbl)
                n883 = Replace Array Subset(array=w1711, new element=w1722, index (row)=12, index (col)=w1704) -> (w1726:string[][])
                n884 = Number To Decimal String(number=w1730) -> (decimal integer string=w1729:string)  [unwired: 1 in]
                n885 = Number To Fractional String(number=w1732) -> (F-format string=w1733:string)  [unwired: 3 in]
                n886 = Number To Decimal String(number=w1732) -> (decimal integer string=w1731:string)  [unwired: 1 in]
                n887 = Array Subset(array=w1711, index (row)=0, index (col)=0) -> (w1717:string[][])  [unwired: 2 in]
                n888 = Index Array(array=w1713, index=0) -> (element=w1712:i32)
                n889 = local read "Index"() -> (w1735:string)
                n890 = Reshape Array(w1717, w1712) -> (w1705:string[])
                n891 = Strip Path(path=w1719) -> (stripped path=w1740:path)  [unwired: 1 out]
                n892 = call "Build Text"("Temp"=w1695, "Index"=w1735, "Length"=w1729, "Width"=w1731) -> ("Result"=w1736:string)  [unwired: 10 in, 1 out]
                n893 = Search 1D Array(1D array=w1705, element=w1699) -> (index of element=w1710:i32)  [unwired: 1 in]
                n894 = Search 1D Array(1D array=w1705, element=w1700) -> (index of element=w1709:i32)  [unwired: 1 in]
                n895 = Replace Array Subset(array=w1726, new element=w1733, index (row)=13, index (col)=w1704) -> (w1728:string[][])
                n896 = Path To String(path=w1740) -> (string=w1738:string)
                n897 = local read "New: Dielectric"() -> (w1742:dbl)
                n898 = Number To Fractional String(number=w1741) -> (F-format string=w1720:string)  [unwired: 3 in]
                n899 = Equal?(x=w1710, y=w1706) -> (x = y?=w1708:bool)
                n900 = Equal?(x=w1709, y=w1706) -> (x = y?=w1707:bool)
                n901 = Replace Array Subset(array=w1728, new element=w1720, index (row)=15, index (col)=w1704) -> (w1727:string[][])
                n902 = Number To Fractional String(number=w1742) -> (F-format string=w1721:string)  [unwired: 3 in]
                n903 = Concatenate Strings(w1738, "\\", w1736) -> (w1737:string)
                n904 = String To Path(string=w1737) -> (path=w1718:path)
                n905 = Replace Array Subset(array=w1727, new element=w1721, index (row)=7, index (col)=w1704) -> (w1703:string[][])
                n906 = case shown="True" w1707 {
                  tunnel: w1709 -> [_ _]
                  tunnel: w1703 -> [w1820 w1828]
                  tunnel: [w1819 w1827] -> w1702
                  tunnel: w1700 -> [_ w1826]
                  frame False {
                    n907 = local read "New: VT-Sat"() -> (w1822:dbl)
                    n908 = Number To Fractional String(number=w1822) -> (F-format string=w1818:string)  [unwired: 3 in]
                    n909 = Replace Array Subset(array=w1820, new element=w1818, index (row)=17, index (col)=1) -> (w1819:string[][])
                  }
                  frame True {
                    n910 = local read "New: VT-Sat"() -> (w1829:dbl)
                    n911 = Number To Fractional String(number=w1829) -> (F-format string=w1825:string)  [unwired: 3 in]
                    n912 = Build Array(w1826, w1825) -> (w1824:string[])
                    n913 = Insert Into Array(array=w1828, index (row)=17, new element=w1824) -> (w1827:string[][])  [unwired: 1 in]
                  }
                }
                n914 = case shown="True" w1708 {
                  tunnel: w1710 -> [_ _]
                  tunnel: w1702 -> [w1807 w1815]
                  tunnel: [w1806 w1814] -> w1701
                  tunnel: w1699 -> [_ w1812]
                  frame False {
                    n915 = local read "New: STS"() -> (w1809:dbl)
                    n916 = Number To Fractional String(number=w1809) -> (F-format string=w1805:string)  [unwired: 3 in]
                    n917 = Replace Array Subset(array=w1807, new element=w1805, index (row)=18, index (col)=1) -> (w1806:string[][])
                  }
                  frame True {
                    n918 = local read "New: STS"() -> (w1816:dbl)
                    n919 = Number To Fractional String(number=w1816) -> (F-format string=w1813:string)  [unwired: 3 in]
                    n920 = Build Array(w1812, w1813) -> (w1811:string[])
                    n921 = Insert Into Array(array=w1815, index (row)=18, new element=w1811) -> (w1814:string[][])  [unwired: 1 in]
                  }
                }
              }
              frame #1 {
                n922 = Equal?(x=w1833, y=w1832) -> (x = y?=w1831:bool)
                n923 = case shown="False" w1831 {
                  tunnel: w1833 -> [w1837 _]
                  tunnel: w1832 -> [w1836 _]
                  frame False {
                    n924 = Move(source path=w1837, 9:TRUE, 10:w1836) -> ()  [unwired: 2 in, 3 out]
                  }
                  frame True {
                  }
                }
              }
              frame #2 {
                n925 = local write "Data File"(w1839) -> ()
                n926 = call-poly <vilib>:"Write To Spreadsheet File.vi"("2D data"=w1838, "file path (dialog if empty)"=w1839) -> ()  [unwired: 6 in, 1 out]
              }
            }
          }
          event "Save Changes? 2": Mouse Down {
            n927 = event-data() -> ()  [unwired: 1 in, 5 out]
            n928 = local read "Data File"() -> (w1863:path)
            n929 = call "Recorded Values.vi"("Path"=w1863) -> ("Recorded Char"=w1861:T5, "Recorded Prop"=w1860:T6, "Fabrication Prop"=w1862:T7)  [unwired: 8 in]
            n930 = Unbundle By Name(w1861) -> ("Mobility-Sat"=w1847:dbl, "Moblitity-Lin"=w1846:dbl, "On/Off"=w1845:dbl, "Threshold Voltage"=w1844:dbl, "STS"=w1843:dbl, "Trap Density-VT"=w1842:dbl, "Trap Density-STS"=w1841:dbl)  [unwired: 1 out]
            n931 = Unbundle By Name(w1860) -> ("Date Recorded"=w1852:string, "Index"=w1851:string, "Length"=w1850:dbl, "Width"=w1849:dbl, "Sample Temp"=w1848:dbl)
            n932 = Unbundle By Name(w1862) -> ("Date Created"=w1840:string, "Material"=w1859:string, "Solvent"=w1858:string, "Concentration"=w1857:dbl, "Method"=w1856:string, "Dielectric (nm)"=w1855:dbl, "Treatment"=w1854:string, "Comments"=w1853:string)
            n933 = local write "Rec: VT-Sat"(w1844) -> ()
            n934 = local write "Date Created"(w1840) -> ()
            n935 = local write "Rec: Material"(w1859) -> ()
            n936 = local write "Rec: Solvent"(w1858) -> ()
            n937 = local write "Rec: Concentration"(w1857) -> ()
            n938 = local write "Rec: Method"(w1856) -> ()
            n939 = local write "Rec: Dielectric (d)"(w1855) -> ()
            n940 = local write "Surface Treatment:"(w1854) -> ()
            n941 = local write "Comments"(w1853) -> ()
            n942 = local write "Index"(w1851) -> ()
            n943 = local write "Rec: Mobility-Sat"(w1847) -> ()
            n944 = local write "Rec: Mobility-Lin"(w1846) -> ()
            n945 = local write "Rec: On/Off"(w1845) -> ()
            n946 = local write "Rec: STS"(w1843) -> ()
            n947 = local write "Rec: Trap Density-VT"(w1842) -> ()
            n948 = local write "Rec: Trap Density-STS"(w1841) -> ()
            n949 = local write "Date Recorded"(w1852) -> ()
            n950 = local write "Rec: Length"(w1850) -> ()
            n951 = local write "Rec: Width"(w1849) -> ()
            n952 = local write "Rec: Temp"(w1848) -> ()
            n953 = stacked-sequence {
              seq-local: [w1943 _ _ _ _] -> [_ w2002 _ _ _]
              seq-local: [w1942 _ _ _ _] -> [_ w2003 _ _ _]
              seq-local: [w1942 _ _ _ _] -> [_ w2001 _ _ _]
              seq-local: [w1925 _ _ _ _] -> [_ w1999 _ _ _]
              seq-local: [_ w2003 _ _ _] -> [_ _ w2008 _ _]
              seq-local: [_ w1999 _ _ _] -> [_ _ w2007 _ _]
              frame #0 {
                w1930 = -1
                w1923 = "STS (V/decade):"
                w1924 = "Threshold V (V):"
                (unwired) 3
                w1928 = 1
                n954 = local read "Rec: Temp"() -> (w1922:dbl)
                n955 = local read "New: Length"() -> (w1954:dbl)
                n956 = local read "Data File"() -> (w1943:path)
                n957 = Equal To 0?(x=w1922) -> (x = 0?=w1921:bool)
                n958 = case shown="False" w1921 {
                  tunnel: [w1968 ""] -> w1920
                  frame False {
                    n959 = local read "Rec: Temp"() -> (w1971:dbl)
                    n960 = Number To Decimal String(number=w1971) -> (decimal integer string=w1970:string)  [unwired: 1 in]
                    n961 = Concatenate Strings("_", w1970, "K") -> (w1968:string)
                  }
                  frame True {
                  }
                }
                n962 = call-poly <vilib>:"Read From Spreadsheet File.vi"("file path (dialog if empty)"=w1943) -> ("all rows"=w1935:string[][])  [unwired: 6 in, 4 out]
                n963 = Number To Fractional String(number=w1954) -> (F-format string=w1946:string)  [unwired: 3 in]
                n964 = local read "New: Width"() -> (w1956:dbl)
                n965 = local read "New: Mobility-Sat"() -> (w1965:dbl)
                n966 = Replace Array Subset(array=w1935, new element=w1946, index (row)=12, index (col)=w1928) -> (w1950:string[][])
                n967 = Number To Fractional String(number=w1956) -> (F-format string=w1957:string)  [unwired: 3 in]
                n968 = Number To Decimal String(number=w1954) -> (decimal integer string=w1953:string)  [unwired: 1 in]
                n969 = Number To Decimal String(number=w1956) -> (decimal integer string=w1955:string)  [unwired: 1 in]
                n970 = local read "Index"() -> (w1959:string)
                n971 = Strip Path(path=w1943) -> (stripped path=w1964:path)  [unwired: 1 out]
                n972 = call "Build Text2"("Temp"=w1920, "Index"=w1959, "Length"=w1953, "Width"=w1955) -> ("Result"=w1960:string)  [unwired: 10 in, 1 out]
                n973 = Replace Array Subset(array=w1950, new element=w1957, index (row)=13, index (col)=w1928) -> (w1952:string[][])
                n974 = Array Size(array=w1935) -> (size(s)=w1937:i32[])
                n975 = Path To String(path=w1964) -> (string=w1962:string)
                n976 = Number To Fractional String(number=w1965) -> (F-format string=w1944:string)  [unwired: 3 in]
                n977 = local read "New: Dielectric"() -> (w1966:dbl)
                n978 = Array Subset(array=w1935, index (row)=0, index (col)=0) -> (w1941:string[][])  [unwired: 2 in]
                n979 = Index Array(array=w1937, index=0) -> (element=w1936:i32)
                n980 = Replace Array Subset(array=w1952, new element=w1944, index (row)=15, index (col)=w1928) -> (w1951:string[][])
                n981 = Number To Fractional String(number=w1966) -> (F-format string=w1945:string)  [unwired: 3 in]
                n982 = Reshape Array(w1941, w1936) -> (w1929:string[])
                n983 = Concatenate Strings(w1962, "\\", w1960) -> (w1961:string)
                n984 = String To Path(string=w1961) -> (path=w1942:path)
                n985 = Search 1D Array(1D array=w1929, element=w1924) -> (index of element=w1933:i32)  [unwired: 1 in]
                n986 = Search 1D Array(1D array=w1929, element=w1923) -> (index of element=w1934:i32)  [unwired: 1 in]
                n987 = Equal?(x=w1933, y=w1930) -> (x = y?=w1931:bool)
                n988 = Equal?(x=w1934, y=w1930) -> (x = y?=w1932:bool)
                n989 = Replace Array Subset(array=w1951, new element=w1945, index (row)=7, index (col)=w1928) -> (w1927:string[][])
                n990 = case shown="False" w1931 {
                  tunnel: w1933 -> [_ _]
                  tunnel: w1927 -> [w1989 w1997]
                  tunnel: [w1988 w1996] -> w1926
                  tunnel: w1924 -> [_ w1995]
                  frame False {
                    n991 = local read "New: VT-Sat"() -> (w1991:dbl)
                    n992 = Number To Fractional String(number=w1991) -> (F-format string=w1987:string)  [unwired: 3 in]
                    n993 = Replace Array Subset(array=w1989, new element=w1987, index (row)=17, index (col)=1) -> (w1988:string[][])
                  }
                  frame True {
                    n994 = local read "New: VT-Sat"() -> (w1998:dbl)
                    n995 = Number To Fractional String(number=w1998) -> (F-format string=w1994:string)  [unwired: 3 in]
                    n996 = Build Array(w1995, w1994) -> (w1993:string[])
                    n997 = Insert Into Array(array=w1997, index (row)=17, new element=w1993) -> (w1996:string[][])  [unwired: 1 in]
                  }
                }
                n998 = case shown="False" w1932 {
                  tunnel: w1934 -> [_ _]
                  tunnel: w1926 -> [w1976 w1984]
                  tunnel: [w1975 w1983] -> w1925
                  tunnel: w1923 -> [_ w1981]
                  frame False {
                    n999 = local read "New: STS"() -> (w1978:dbl)
                    n1000 = Number To Fractional String(number=w1978) -> (F-format string=w1974:string)  [unwired: 3 in]
                    n1001 = Replace Array Subset(array=w1976, new element=w1974, index (row)=18, index (col)=1) -> (w1975:string[][])
                  }
                  frame True {
                    n1002 = local read "New: STS"() -> (w1985:dbl)
                    n1003 = Number To Fractional String(number=w1985) -> (F-format string=w1982:string)  [unwired: 3 in]
                    n1004 = Build Array(w1981, w1982) -> (w1980:string[])
                    n1005 = Insert Into Array(array=w1984, index (row)=18, new element=w1980) -> (w1983:string[][])  [unwired: 1 in]
                  }
                }
              }
              frame #1 {
                n1006 = Equal?(x=w2002, y=w2001) -> (x = y?=w2000:bool)
                n1007 = case shown="False" w2000 {
                  tunnel: w2002 -> [w2006 _]
                  tunnel: w2001 -> [w2005 _]
                  frame False {
                    n1008 = Move(source path=w2006, 9:TRUE, 10:w2005) -> ()  [unwired: 2 in, 3 out]
                  }
                  frame True {
                  }
                }
              }
              frame #2 {
                n1009 = local write "Data File"(w2008) -> ()
                n1010 = call-poly <vilib>:"Write To Spreadsheet File.vi"("2D data"=w2007, "file path (dialog if empty)"=w2008) -> ()  [unwired: 6 in, 1 out]
              }
              frame #3 {
                w2066 = 0
                # "Moves to next file and displays new image/data"
                n1011 = property on="Image Out" class="ImageControl"() -> (error out=w2028:errorcluster, "Image Center Position"=w2032:cluster{"X":u32, "Y":u32})  [unwired: 2 in, 1 out]
                n1012 = local read "Data File"() -> (w2071:path)
                n1013 = Strip Path(path=w2071) -> (stripped path=w2062:path, name=w2080:string)
                n1014 = Unbundle(w2032) -> ("X"=w2030:u32)  [unwired: 1 out]
                n1015 = local write "Data Folder"(w2062) -> ()
                n1016 = Bundle("X"=w2030, 0) -> (w2031:cluster{"X":u32, i32})  [unwired: 1 in]
                n1017 = property on="Image Out" class="ImageControl"(error in=w2028, "Image Center Position"=w2031) -> ()  [unwired: 1 in, 2 out]
                n1018 = List Folder(path=w2062) -> (filenames=w2076:string[])  [unwired: 3 in, 3 out]
                n1019 = Search 1D Array(1D array=w2076, element=w2080) -> (index of element=w2073:i32)  [unwired: 1 in]
                n1020 = Array Size(array=w2076) -> (size(s)=w2072:i32)
                n1021 = Decrement(x=w2072) -> (x-1=w2074:i32)
                n1022 = Equal?(x=w2073, y=w2074) -> (x = y?=w2075:bool)
                n1023 = local read "Folder Index"() -> (w2024:dbl)
                n1024 = case shown="False" w2075 {
                  tunnel: w2024 -> [w2203 _]
                  tunnel: [w2202 0] -> w2023
                  frame False {
                    n1025 = Increment(x=w2203) -> (x+1=w2202:dbl)
                  }
                  frame True {
                  }
                }
                n1026 = invoke on="Image Out" class="ImageControl" method="Clear ROI"() -> ()  [unwired: 3 in, 3 out]
                n1027 = local write "Folder Index"(w2023) -> ()
                n1028 = Path To String(path=w2062) -> (string=w2081:string)
                n1029 = Index Array(array=w2076, index=w2023) -> (element=w2077:string)
                n1030 = local write "Data Name:"(w2077) -> ()
                n1031 = Concatenate Strings(w2081, "\\", w2077) -> (w2079:string)
                n1032 = String To Path(string=w2079) -> (path=w2022:path)
                n1033 = local write "Data File"(w2022) -> ()
                n1034 = local read "NumPts 2"() -> (w2013:dbl)
                n1035 = local read "NumPts"() -> (w2014:dbl)
                n1036 = call-poly <vilib>:"Read From Spreadsheet File.vi"("file path (dialog if empty)"=w2022) -> ("all rows"=w2068:string[][])  [unwired: 6 in, 4 out]
                n1037 = call "Mobility-Vt Calculator-File.vi"("NumPts"=w2014, "Path"=w2022) -> ("XY Graph-Sat"=w2016:cluster{dbl[], dbl[]}[], "Output"=w2017:T8, "Index-Sat"=w2015:dbl)  [unwired: 4 in, 3 out]
                n1038 = call "STS Calculator-File.vi"("NumPts"=w2013, "Path"=w2022) -> ("STS Index-Sat"=w2012:dbl, "XY Graph-Sat"=w2011:cluster{dbl[], dbl[]}[], "Ouput"=w2010:cluster{"STS-Sat":dbl, "STS-Lin":dbl})  [unwired: 5 in, 2 out]
                n1039 = local write "MobVi Index"(w2015) -> ()
                n1040 = local write "Slide"(w2015) -> ()
                n1041 = local write "XY Graph"(w2016) -> ()
                n1042 = local write "Index 2"(w2012) -> ()
                n1043 = local write "XY Graph 2"(w2011) -> ()
                n1044 = Unbundle By Name(w2017) -> ("Mobility-Sat"=w2021:dbl, "Vt-Sat"=w2020:dbl, "Mobility-Lin"=w2019:dbl, "Mobility-Lin"=w2018:dbl)
                n1045 = Array Size(array=w2068) -> (size(s)=w2067:i32[])
                n1046 = Unbundle By Name(w2010) -> ("STS-Sat"=w2009:dbl)
                n1047 = local write "Calc: Mobility-Sat"(w2021) -> ()
                n1048 = local write "Calc: Mobility-Lin"(w2018) -> ()
                n1049 = local read "Image Folder"() -> (w2056:path)
                n1050 = local write "Calc: VT-Sat"(w2020) -> ()
                n1051 = local write "Calc: VT-Lin"(w2019) -> ()
                n1052 = Decimate 1D Array(w2016) -> (w2051:cluster{dbl[], dbl[]}[])  [unwired: 1 out]
                n1053 = Index Array(array=w2067, index=w2066) -> (element=w2047:i32)
                n1054 = Decimate 1D Array(w2011) -> (w2041:cluster{dbl[], dbl[]}[])  [unwired: 1 out]
                n1055 = Array Subset(array=w2068, index (row)=w2066, index (col)=w2066, length (col)=3) -> (w2069:string[][])  [unwired: 1 in]
                n1056 = local write "Calc: STS"(w2009) -> ()
                n1057 = List Folder(path=w2056) -> (filenames=w2061:string[])  [unwired: 3 in, 3 out]
                n1058 = Array To Cluster(array=w2051) -> (cluster=w2053:T9)
                n1059 = Array To Cluster(array=w2041) -> (cluster=w2039:T9)
                n1060 = Reshape Array(w2069, w2047) -> (w2054:string[])
                n1061 = Subtract(x=w2047, y=20) -> (x-y=w2046:i32)
                n1062 = property on="Slide" class="Slide (strict)"("Scale.Maximum"=w2046) -> ()  [unwired: 2 in, 2 out]
                n1063 = Unbundle(w2053) -> ("[0]"=w2052:cluster{dbl[], dbl[]})  [unwired: 8 out]
                n1064 = Unbundle(w2039) -> ("[0]"=w2040:cluster{dbl[], dbl[]})  [unwired: 8 out]
                n1065 = Search 1D Array(1D array=w2054, element="Index:") -> (index of element=w2063:i32)  [unwired: 1 in]
                n1066 = Increment(x=w2063) -> (x+1=w2064:i32)
                n1067 = Unbundle(w2052) -> (w2043:dbl[], w2042:dbl[])
                n1068 = Unbundle(w2040) -> (w2038:dbl[], w2037:dbl[])
                n1069 = Array Subset(array=w2043, index=w2015, length=w2014) -> (w2050:dbl[])
                n1070 = Array Subset(array=w2042, index=w2015, length=w2014) -> (w2049:dbl[])
                n1071 = Array Subset(array=w2038, index=w2012, length=w2013) -> (w2045:dbl[])
                n1072 = Array Subset(array=w2037, index=w2012, length=w2013) -> (w2044:dbl[])
                n1073 = Index Array(array=w2054, index=w2064) -> (element=w2059:string)
                n1074 = local write "Sat Vg Array-Used"(w2050) -> ()
                n1075 = local write "Vg Array-Log-Used"(w2044) -> ()
                n1076 = local write "Sat Id-Log-Used"(w2045) -> ()
                n1077 = local write "Sat Id-Used"(w2049) -> ()
                n1078 = local write "Index"(w2059) -> ()
                n1079 = while {
                  tunnel: w2061 -> [w2089]
                  tunnel: w2059 -> [w2087]
                  tunnel: [w2086] -> _
                  tunnel: [w2086] -> w2060
                  tunnel: w2047 -> [w2085]
                  i -> [w2086]
                  stop <- w2082 stop-if-true
                  n1080 = Index Array(array=w2089, index=w2086) -> (element=w2090:string)
                  n1081 = xnode "Match Regular Expression"("input string"=w2090, "regular expression"=w2087) -> ("whole match"=w2088:string)  [unwired: 4 in, 4 out]
                  n1082 = Equal?(x=w2088, y=w2087) -> (x = y?=w2084:bool)
                  n1083 = Equal?(x=w2085, y=w2086) -> (x = y?=w2083:bool)
                  n1084 = Or(x=w2084, y=w2083) -> (x .or. y?=w2082:bool)
                }
                n1085 = Path To String(path=w2056) -> (string=w2058:string)
                n1086 = Index Array(array=w2061, index=w2060) -> (element=w2035:string)
                n1087 = local write "Image Name"(w2035) -> ()
                n1088 = Empty String/Path?(string/path=w2035) -> (empty?=w2036:bool)
                n1089 = Concatenate Strings(w2058, "\\", w2035) -> (w2057:string)
                n1090 = String To Path(string=w2057) -> (path=w2034:path)
                n1091 = local read "No Image"() -> (w2033:path)
                n1092 = Select(t=w2033, s=w2036, f=w2034) -> (s? t:f=w2027:path)
                n1093 = local write "Image File"(w2027) -> ()
                n1094 = local read "Image Out"() -> (w2025:T2)
                n1095 = call "IMAQ ReadFile"("File Path"=w2027, "Image"=w2025) -> ("Image Out"=w2026:T2)  [unwired: 5 in, 4 out]
                n1096 = local write "Image Out"(w2026) -> ()
                n1097 = local write "Image Out 2"(w2026) -> ()
              }
              frame #4 {
                # "Output ROI data"
                n1098 = local read "Image Folder"() -> (w2205:path)
                n1099 = Build Path(base path=w2205, name or relative path="ROI") -> (appended path=w2207:path)
                n1100 = local read "Index"() -> (w2206:string)
                n1101 = Build Path(base path=w2207, name or relative path=w2206) -> (appended path=w2212:path)
                n1102 = invoke on="Image Out" class="ImageControl" method="Clear ROI"() -> (error out=w2211:errorcluster)  [unwired: 3 in, 2 out]
                n1103 = call <vilib>:"Check if File or Folder Exists.vi"("error in (no error)"=w2211, "path"=w2212) -> ("file or folder exists?"=w2209:bool, "dup path"=w2210:path)  [unwired: 7 in, 1 out]
                n1104 = case shown="True" w2209 {
                  tunnel: w2210 -> [_ w2213]
                  frame False {
                  }
                  frame True {
                    n1105 = Read from Text File(file (use dialog)=w2213) -> (text=w2217:string)  [unwired: 3 in, 3 out]
                    n1106 = property on="Image Out" class="ImageControl"() -> ("ROI"=w2214:T10)  [unwired: 2 in, 2 out]
                    n1107 = Unflatten From String(type=w2214, binary string=w2217) -> (value=w2215:T10, error out=w2216:errorcluster)  [unwired: 3 in, 1 out]
                    n1108 = property on="Image Out" class="ImageControl"(error in=w2216, "ROI"=w2215) -> ()  [unwired: 1 in, 2 out]
                  }
                }
              }
            }
            n1109 = flat-sequence {
              tunnel: [w1877] -> w1864
              tunnel: w1864 -> [w1891]
              frame #0 {
                # "Makes Empty File for Transformer Data"
                n1110 = local read "Data Folder"() -> (w1866:path)
                n1111 = Build Path(base path=w1866, name or relative path="Stats") -> (appended path=w1868:path)
                n1112 = call <vilib>:"Check if File or Folder Exists.vi"("path"=w1868) -> ("file or folder exists?"=w1869:bool, "dup path"=w1870:path)  [unwired: 8 in, 1 out]
                n1113 = case shown="False" w1869 {
                  tunnel: [w1874 w1876] -> w1871
                  tunnel: w1870 -> [w1875 w1876]
                  frame False {
                    n1114 = Create Folder(path (use dialog)=w1875) -> (created path=w1874:path)  [unwired: 2 in, 2 out]
                  }
                  frame True {
                  }
                }
                n1115 = Build Path(base path=w1871, name or relative path="Tranformer Data.txt") -> (appended path=w1873:path)
                n1116 = call-poly <vilib>:"Write To Spreadsheet File.vi"("append to file? (new file:F)"=TRUE, "file path (dialog if empty)"=w1873) -> ()  [unwired: 6 in, 1 out]
              }
              frame #1 {
                # "Adds Headers if they don't exist"
                n1117 = Concatenate Strings("Stats\\", "Tranformer Data.txt") -> (w1884:string)
                n1118 = local read "Data Folder"() -> (w1883:path)
                n1119 = Build Path(base path=w1883, name or relative path=w1884) -> (appended path=w1877:path)
                n1120 = call-poly <vilib>:"Read From Spreadsheet File.vi"("file path (dialog if empty)"=w1877) -> ("first row"=w1882:string[])  [unwired: 6 in, 4 out]
                n1121 = Search 1D Array(1D array=w1882, element="DeviceID") -> (index of element=w1880:i32)  [unwired: 1 in]
                n1122 = Equal?(x=w1880, y=0) -> (x = y?=w1878:bool)
                n1123 = case shown="False" w1878 {
                  tunnel: w1877 -> [w1888 _]
                  frame False {
                    n1124 = local read "Transformer \nHeaders"() -> (w1887:string[])
                    n1125 = call-poly <vilib>:"Write To Spreadsheet File.vi"("1D data"=w1887, "file path (dialog if empty)"=w1888) -> ()  [unwired: 6 in, 1 out]
                  }
                  frame True {
                  }
                }
              }
              frame #2 {
                # "Adds current device if it doesn't exist"
                n1126 = local read "Current \nRecord"() -> (w1894:string[])
                n1127 = Index Array(array=w1894, index=0) -> (element=w1893:string)
                n1128 = Concatenate Strings("Stats\\", "Tranformer Data.txt") -> (w1897:string)
                n1129 = local read "Data Folder"() -> (w1896:path)
                n1130 = local write "Current Device ID"(w1893) -> ()
                n1131 = local read "Current Device ID"() -> (w1903:string)
                n1132 = Build Path(base path=w1896, name or relative path=w1897) -> (appended path=w1895:path)
                n1133 = call-poly <vilib>:"Read From Spreadsheet File.vi"("file path (dialog if empty)"=w1895) -> ("all rows"=w1890:string[][])  [unwired: 6 in, 4 out]
                n1134 = Index Array(array=w1890, index (col)=0) -> (element=w1901:string[])  [unwired: 1 in]
                n1135 = Search 1D Array(1D array=w1901, element=w1903) -> (index of element=w1889:i32)  [unwired: 1 in]
                n1136 = Equal?(x=w1889, y=-1) -> (x = y?=w1892:bool)
                n1137 = case shown="False" w1892 {
                  tunnel: w1891 -> [w1905 w1918]
                  tunnel: w1889 -> [w1910 _]
                  tunnel: w1890 -> [w1911 _]
                  frame False {
                    n1138 = local read "Current \nRecord"() -> (w1909:string[])
                    n1139 = Replace Array Subset(array=w1911, new element=w1909, index (row)=w1910) -> (w1906:string[][])  [unwired: 1 in]
                    n1140 = flat-sequence {
                      tunnel: [w1912] -> _
                      tunnel: [w1913] -> _
                      tunnel: [w1913] -> w1908
                      tunnel: [w1912] -> w1907
                      tunnel: w1906 -> [w1913]
                      tunnel: w1905 -> [w1912]
                      tunnel: w1908 -> [w1915]
                      tunnel: w1907 -> [w1914]
                      frame #0 {
                        n1141 = Delete(path (use dialog)=w1912) -> ()  [unwired: 4 in, 3 out]
                      }
                      frame #1 {
                        n1142 = call-poly <vilib>:"Write To Spreadsheet File.vi"("append to file? (new file:F)"=TRUE, "2D data"=w1915, "file path (dialog if empty)"=w1914) -> ()  [unwired: 5 in, 1 out]
                      }
                    }
                  }
                  frame True {
                    n1143 = local read "Current \nRecord"() -> (w1917:string[])
                    n1144 = call-poly <vilib>:"Write To Spreadsheet File.vi"("append to file? (new file:F)"=TRUE, "1D data"=w1917, "file path (dialog if empty)"=w1918) -> ()  [unwired: 5 in, 1 out]
                  }
                }
              }
            }
          }
          event "Export": Mouse Down {
            n1145 = event-data() -> ()  [unwired: 1 in, 7 out]
            n1146 = call "OA_ConnectToOrigin.vi"() -> ("error out"=w2239:errorcluster, "Origin.IOApplication"=w2240:refnum<k7>)  [unwired: 8 in]
            n1147 = local read "Data Folder"() -> (w2218:path)
            n1148 = local read "Project"() -> (w2238:path)
            n1149 = call "OA_Load.vi"("error in (no error)"=w2239, "Path"=w2238, "Origin.IOApplication"=w2240) -> ("error out"=w2231:errorcluster, "Origin.IOApplication"=w2232:refnum<k7>)  [unwired: 1 out]
            n1150 = call "OAExecute.vi"("script"="document -m 3;", "Error IO"=w2231, "Origin.IOApplication"=w2232) -> ("Error IO Out"=w2229:errorcluster, "Origin.IOApplication"=w2230:refnum<k7>)  [unwired: 1 in, 1 out]
            n1151 = Build Path(base path=w2218, name or relative path="Stats") -> (appended path=w2219:path)
            n1152 = flat-sequence {
              tunnel: w2218 -> [w2260]
              tunnel: w2237 -> [w2259]
              tunnel: [w2249] -> w2242
              tunnel: [w2250] -> w2241
              tunnel: w2230 -> [w2254]
              tunnel: w2229 -> [w2253]
              tunnel: w2218 -> [w2276]
              tunnel: w2237 -> [w2275]
              tunnel: w2242 -> [w2271]
              tunnel: w2241 -> [w2272]
              tunnel: [w2266] -> w2236
              tunnel: [w2265] -> w2235
              tunnel: w2218 -> [w2287]
              tunnel: w2237 -> [w2286]
              tunnel: w2236 -> [w2282]
              tunnel: w2235 -> [w2281]
              tunnel: [w2280] -> w2234
              tunnel: [w2279] -> w2233
              tunnel: w2218 -> [w2302]
              tunnel: w2237 -> [w2301]
              tunnel: w2234 -> [w2296]
              tunnel: w2233 -> [w2295]
              tunnel: [w2293] -> w2227
              tunnel: [w2292] -> w2226
              frame #0 {
                n1153 = call "Param_Analysis.vi"("error in (no error)"=w2253, "Folder 2"=w2260, "Parameter String"="Mobility (cm^2/Vs):", "Parameter Name"="Mobility", "Folder"=w2259) -> ("error out"=w2256:errorcluster, "Array 4"=w2246:string[], "Array 3"=w2255:string[][])  [unwired: 3 in, 1 out]
                n1154 = call "Origin_Export.vi"("String 3"="[MobHistTab]Sheet1", "error in (no error)"=w2256, "Array"=w2255, "String 2"="[MOBvsLTable]Mobilities", "String"="pe_cd \"Mobility Chart\";", "Origin.IOApplication"=w2254, "Array 2"=w2246) -> ("reference out"=w2252:refnum<k7>, "error out"=w2251:errorcluster)  [unwired: 2 in, 1 out]
                n1155 = call "OAExecute.vi"("script"="window -a MOBvsLTable;\nwindow -s TV;", "Error IO"=w2251, "Origin.IOApplication"=w2252) -> ("Error IO Out"=w2249:errorcluster, "Origin.IOApplication"=w2250:refnum<k7>)  [unwired: 1 in, 1 out]
              }
              frame #1 {
                n1156 = call "Param_Analysis.vi"("error in (no error)"=w2271, "Folder 2"=w2276, "Parameter String"="On/Off Current:", "Parameter Name"="On_Off_Current", "Folder"=w2275) -> ("error out"=w2270:errorcluster, "Array 4"=w2264:string[], "Array 3"=w2267:string[][])  [unwired: 3 in, 1 out]
                n1157 = call "Origin_Export.vi"("String 3"="[OnOffHistTab]Sheet1", "error in (no error)"=w2270, "Array"=w2267, "String 2"="[OnOffTable]On/Off Ratios", "String"="pe_cd \"OnOff vs L\";", "Origin.IOApplication"=w2272, "Array 2"=w2264) -> ("reference out"=w2266:refnum<k7>, "error out"=w2265:errorcluster)  [unwired: 2 in, 1 out]
              }
              frame #2 {
                n1158 = call "Param_Analysis.vi"("Folder 2"=w2287, "Parameter String"="S.T.S. (V/decade):", "Parameter Name"="STS", "Folder"=w2286) -> ("Array 4"=w2278:string[], "Array 3"=w2283:string[][])  [unwired: 4 in, 2 out]
                n1159 = call "Origin_Export.vi"("String 3"="[SHistTab]Sheet1", "error in (no error)"=w2281, "Array"=w2283, "String 2"="[STable]Threshold Swing", "String"="pe_cd \"Threshold Swing vs L\";", "Origin.IOApplication"=w2282, "Array 2"=w2278) -> ("reference out"=w2279:refnum<k7>, "error out"=w2280:errorcluster)  [unwired: 2 in, 1 out]
              }
              frame #3 {
                n1160 = call "Param_Analysis.vi"("Folder 2"=w2302, "Parameter String"="Threshold V (V):", "Parameter Name"="Threshold_V", "Folder"=w2301) -> ("Array 4"=w2291:string[], "Array 3"=w2294:string[][])  [unwired: 4 in, 2 out]
                n1161 = call "Origin_Export.vi"("String 3"="[VtHistTab]Sheet1", "error in (no error)"=w2296, "Array"=w2294, "String 2"="[VtTable]Threshold Voltages", "String"="pe_cd \"Threshold Voltage vs L\";", "Origin.IOApplication"=w2295, "Array 2"=w2291) -> ("reference out"=w2293:refnum<k7>, "error out"=w2292:errorcluster)  [unwired: 2 in, 1 out]
              }
            }
            n1162 = call <vilib>:"Check if File or Folder Exists.vi"("path"=w2219) -> ("file or folder exists?"=w2244:bool, "dup path"=w2243:path)  [unwired: 8 in, 1 out]
            n1163 = case shown="False" w2244 {
              tunnel: w2243 -> [w2304 w2305]
              tunnel: [w2303 w2305] -> w2237
              frame False {
                n1164 = Create Folder(path (use dialog)=w2304) -> (created path=w2303:path)  [unwired: 2 in, 2 out]
              }
              frame True {
              }
            }
            n1165 = call "File Dialog"("start path"=w2219) -> ("selected path"=w2222:path)  [unwired: 11 in, 3 out]
            n1166 = Path To String(path=w2222) -> (string=w2221:string)
            n1167 = call "OAExecute.vi"("script"="pe_cd /;\npe_cd \"Mobility Chart\"; ", "Error IO"=w2226, "Origin.IOApplication"=w2227) -> ("Error IO Out"=w2223:errorcluster, "Origin.IOApplication"=w2224:refnum<k7>)  [unwired: 1 in, 1 out]
            n1168 = call "OASaveProject.vi"("path"=w2221, "Error IO"=w2223, "Origin.IOApplication"=w2224) -> ()  [unwired: 3 out]
          }
          event "Blank Button": Mouse Down {
            n1169 = event-data() -> ()  [unwired: 1 in, 7 out]
            n1170 = local read "Data File"() -> (w2313:path)
            n1171 = Strip Path(path=w2313) -> (stripped path=w2309:path, name=w2311:string)
            n1172 = Path To String(path=w2309) -> (string=w2308:string)
            n1173 = Concatenate Strings(w2308, "\\", "X_", w2311) -> (w2307:string)
            n1174 = String To Path(string=w2307) -> (path=w2306:path)
            n1175 = Move(source path=w2313, 10:w2306) -> ()  [unwired: 3 in, 3 out]
            n1176 = local write "Data File"(w2306) -> ()
          }
          event "Cancel Button": Mouse Down {
            (unwired) 6
            n1177 = event-data() -> ()  [unwired: 1 in, 7 out]
            n1178 = call "Simulate_Keyboard.vi"("Action"=2, "Virtual Key"=162) -> ()  [unwired: 7 in, 1 out]
          }
        }
        n1179 = Reciprocal(x=w512) -> (1/x=w511:sgl)
        n1180 = Multiply(x=w511, y=10) -> (x*y=w513:sgl)
        n1181 = case shown="\"EQUALS\"" w552 {
          tunnel: w526 -> [w605 w611 w615 w617 w621 w623 w625 w627 w629 w631 w633 w635 w637 w639 w641 w643 w645 w647 w649 w651 w653 w655 w657 w659 w661 w663 w665 w667 w669 w671 w673 w675 w677 w679 w681 w683 w685 w687 w689 w691 w693 w695 w697 w699 w701 w703 w705 w707 w709 w711 w713 w715 w717 w719 w721 w723 w725 w727 w729 w731 w733 w735 w737 w739 w741 w743 w745 w747 w749 w751 w753 w755 w757 w759 w761 w763 w765 w767 w769 w771 w773 w775 w777 w779 w781 w783 w785 w787 w789 w791 w793 w795 w797 w799 w801 w803 w805 w807 w809 w811 w813 w815 w817 w819 w821]
          tunnel: [w605 w610 w614 w617 w621 w623 w625 w627 w629 w631 w633 w635 w637 w639 w641 w643 w645 w647 w649 w651 w653 w655 w657 w659 w661 w663 w665 w667 w669 w671 w673 w675 w677 w679 w681 w683 w685 w687 w689 w691 w693 w695 w697 w699 w701 w703 w705 w707 w709 w711 w713 w715 w717 w719 w721 w723 w725 w727 w729 w731 w733 w735 w737 w739 w741 w743 w745 w747 w749 w751 w753 w755 w757 w759 w761 w763 w765 w767 w769 w771 w773 w775 w777 w779 w781 w783 w785 w787 w789 w791 w793 w795 w797 w799 w801 w803 w805 w807 w809 w811 w813 w815 w817 w819 w821] -> w551
          tunnel: w527 -> [w607 w609 w613 w619 w620 w622 w624 w626 w628 w630 w632 w634 w636 w638 w640 w642 w644 w646 w648 w650 w652 w654 w656 w658 w660 w662 w664 w666 w668 w670 w672 w674 w676 w678 w680 w682 w684 w686 w688 w690 w692 w694 w696 w698 w700 w702 w704 w706 w708 w710 w712 w714 w716 w718 w720 w722 w724 w726 w728 w730 w732 w734 w736 w738 w740 w742 w744 w746 w748 w750 w752 w754 w756 w758 w760 w762 w764 w766 w768 w770 w772 w774 w776 w778 w780 w782 w784 w786 w788 w790 w792 w794 w796 w798 w800 w802 w804 w806 w808 w810 w812 w814 w816 w818 w820]
          tunnel: [w606 w609 w613 w618 w620 w622 w624 w626 w628 w630 w632 w634 w636 w638 w640 w642 w644 w646 w648 w650 w652 w654 w656 w658 w660 w662 w664 w666 w668 w670 w672 w674 w676 w678 w680 w682 w684 w686 w688 w690 w692 w694 w696 w698 w700 w702 w704 w706 w708 w710 w712 w714 w716 w718 w720 w722 w724 w726 w728 w730 w732 w734 w736 w738 w740 w742 w744 w746 w748 w750 w752 w754 w756 w758 w760 w762 w764 w766 w768 w770 w772 w774 w776 w778 w780 w782 w784 w786 w788 w790 w792 w794 w796 w798 w800 w802 w804 w806 w808 w810 w812 w814 w816 w818 w820] -> w550
          tunnel: w513 -> [w604 w608 w612 w616 _ _ _ _ _ _ _ _ _ _ _ _ _ _ _ _ _ _ _ _ _ _ _ _ _ _ _ _ _ _ _ _ _ _ _ _ _ _ _ _ _ _ _ _ _ _ _ _ _ _ _ _ _ _ _ _ _ _ _ _ _ _ _ _ _ _ _ _ _ _ _ _ _ _ _ _ _ _ _ _ _ _ _ _ _ _ _ _ _ _ _ _ _ _ _ _ _ _ _ _ _]
          frame "DOWN" {
            n1182 = Add(x=w607, y=w604) -> (x+y=w606:sgl)
          }
          frame "LEFT" {
            n1183 = Subtract(x=w611, y=w608) -> (x-y=w610:sgl)
          }
          frame "RIGHT" {
            n1184 = Add(x=w615, y=w612) -> (x+y=w614:sgl)
          }
          frame "UP" {
            n1185 = Subtract(x=w619, y=w616) -> (x-y=w618:sgl)
          }
          frame "ENTER (num pad)" {
          }
          frame "' (quote)" {
          }
          frame "END" {
          }
          frame "EQUALS" {
          }
          frame "ESCAPE" {
          }
          frame "GRAVE (`)" {
          }
          frame "HOME" {
          }
          frame "INSERT" {
          }
          frame "LBRACKET" {
          }
          frame "LCONTROL" {
          }
          frame "L ALT" {
          }
          frame "LSHIFT" {
          }
          frame "LWIN" {
          }
          frame "MINUS" {
          }
          frame "MULTIPLY" {
          }
          frame "NEXT" {
          }
          frame "NUMLOCK" {
          }
          frame "NUMPAD_0" {
          }
          frame "NUMPAD_1" {
          }
          frame "NUMPAD_2" {
          }
          frame "NUMPAD_3" {
          }
          frame "NUMPAD_4" {
          }
          frame "NUMPAD_5" {
          }
          frame "NUMPAD_6" {
          }
          frame "NUMPAD_7" {
          }
          frame "NUMPAD_8" {
          }
          frame "NUMPAD_9" {
          }
          frame "PAUSE" {
          }
          frame "PERIOD" {
          }
          frame "PRIOR (PG UP)" {
          }
          frame "RBRACKET" {
          }
          frame "RCONTROL" {
          }
          frame "RETURN" {
          }
          frame "R ALT" {
          }
          frame "RSHIFT" {
          }
          frame "RWIN" {
          }
          frame "SCROLL" {
          }
          frame "SEMICOLON" {
          }
          frame "SLASH" {
          }
          frame "SPACE" {
          }
          frame "SUBTRACT" {
          }
          frame "TAB" {
          }
          frame "DIVIDE" {
          }
          frame "DELETE" {
          }
          frame "DECIMAL" {
          }
          frame "COMMA" {
          }
          frame "CAPITAL" {
          }
          frame "BACKSLASH" {
          }
          frame "BACK" {
          }
          frame "ADD" {
          }
          frame "F15" {
          }
          frame "F14" {
          }
          frame "F13" {
          }
          frame "F12" {
          }
          frame "F11" {
          }
          frame "F10" {
          }
          frame "F9" {
          }
          frame "F8" {
          }
          frame "F7" {
          }
          frame "F6" {
          }
          frame "F5" {
          }
          frame "F4" {
          }
          frame "F3" {
          }
          frame "F2" {
          }
          frame "F1" {
          }
          frame "Z" {
          }
          frame "Y" {
          }
          frame "X" {
          }
          frame "W" {
          }
          frame "V" {
          }
          frame "U" {
          }
          frame "T" {
          }
          frame "S" {
          }
          frame "R" {
          }
          frame "Q" {
          }
          frame "P" {
          }
          frame "O" {
          }
          frame "N" {
          }
          frame "M" {
          }
          frame "L" {
          }
          frame "K" {
          }
          frame "J" {
          }
          frame "I" {
          }
          frame "H" {
          }
          frame "G" {
          }
          frame "F" {
          }
          frame "E" {
          }
          frame "D" {
          }
          frame "C" {
          }
          frame "B" {
          }
          frame "A" {
          }
          frame "9" {
          }
          frame "8" {
          }
          frame "7" {
          }
          frame "6" {
          }
          frame "5" {
          }
          frame "4" {
          }
          frame "3" {
          }
          frame "2" {
          }
          frame "1" {
          }
          frame "0" {
          }
        }
        n1186 = Bundle(w529, w528, w543, w542, 0.0) -> (w541:cluster{dbl, dbl, dbl, dbl, dbl})  [unwired: 1 in]
        n1187 = Bundle("X"=w551, "Y"=w550) -> (w545:cluster{"X":sgl, "Y":sgl})  [unwired: 1 in]
        n1188 = Divide(x=20, y=w512) -> (x/y=w515:sgl)
        n1189 = property on="Image Out" class="ImageControl"("Image Center Position"=w545) -> ()  [unwired: 2 in, 2 out]
        n1190 = call "IMAQ Convert Rectangle to ROI (Polygon)"("Rectangle"=w541) -> ("ROI Descriptor"=w539:T3)  [unwired: 7 in, 2 out]
        n1191 = Bundle("Application Font", w515, w519, w519, w519, w519, w519, TRUE, w517) -> (w521:T16)  [unwired: 1 in]
        n1192 = property on="Image Out 2" class="ImageControl"("ROI"=w539) -> ()  [unwired: 2 in, 2 out]
        n1193 = Bundle(w517, w521, w517, w517) -> (w520:T17)  [unwired: 1 in]
        n1194 = property on="Image Out" class="ImageControl"() -> ("ROI"=w504:T10)  [unwired: 2 in, 2 out]
        n1195 = Unbundle By Name(w504) -> ("Contours"=w568:T14)
        n1196 = local read "Image Out"() -> (w523:T2)
        n1197 = call "IMAQ Clear Overlay"("Image"=w523) -> ("Image Out"=w522:T2)  [unwired: 9 in, 1 out]
        n1198 = Initialize Array(0) -> (w566:i32[])  [unwired: 1 in]
        n1199 = local read "Magnification"() -> (w557:u16)
        n1200 = Array Size(array=w568) -> (size(s)=w567:i32)
        n1201 = Build Array(0.505025, 0.252522, 0.127742, 0.050345, 0.031129) -> (w558:dbl[])
        n1202 = Array Subset(array=w558, index=w557, length=1) -> (w555:dbl[])
        n1203 = property on="Image Out" class="ImageControl"() -> ("ZoomInteger"=w547:cluster{"X":i32, "Y":i32})  [unwired: 2 in, 2 out]
        n1204 = To Double Precision Float(number=w555) -> (double precision float=w554:dbl[])
        n1205 = for {
          N: w567 -> [_]
          shift-right: [w844] -> _
          shift-left: w568 -> [w844]
          shift-right: [w842] -> w553
          shift-left: w566 -> [w841]
          tunnel: w554 -> [w840]
          shift-right: [w837] -> _
          shift-left: w522 -> [w839]
          tunnel: w520 -> [w832]
          i -> [w836]
          n1206 = Index Array(array=w844, index=w836) -> (element=w853:T18)
          n1207 = Unbundle(w853) -> ("Points"=w852:i32[])  [unwired: 2 out]
          n1208 = Array To Cluster(array=w852) -> (cluster=w851:T19)
          n1209 = Unbundle(w851) -> ("Points[0]"=w831:i32, "Points[1]"=w828:i32, "Points[2]"=w843:i32, "Points[3]"=w849:i32)  [unwired: 5 out]
          n1210 = Add(x=w831, y=10) -> (x+y=w829:i32)
          n1211 = Subtract(x=w828, y=w849) -> (x-y=w848:i32)
          n1212 = Subtract(x=w831, y=w843) -> (x-y=w850:i32)
          n1213 = Square(x=w848) -> (x^2=w846:i32)
          n1214 = Square(x=w850) -> (x^2=w847:i32)
          n1215 = Add(x=w847, y=w846) -> (x+y=w845:i32)
          n1216 = Square Root(x=w845) -> (sqrt(x)=w822:dbl)
          n1217 = Multiply(x=w822, y=0.5) -> (x*y=w825:dbl)
          n1218 = Add(x=w825, y=w828) -> (x+y=w827:dbl)
          n1219 = Bundle(w829, w827) -> (w838:cluster{i32, dbl})  [unwired: 1 in]
          n1220 = Multiply(x=w822, y=w840) -> (x*y=w835:dbl[])
          n1221 = Index Array(array=w835) -> (element=w834:dbl)  [unwired: 1 in]
          n1222 = Number To Fractional String(number=w834) -> (F-format string=w833:string)  [unwired: 3 in]
          n1223 = call "IMAQ Overlay Text"("BG Color (Transparent)"=u32 0, "Text Color (black)"=u32 16448250, "Font, Size & Style"=w832, "String"=w833, "Origin"=w838, "Image"=w839) -> ("Image Out"=w837:T2)  [unwired: 4 in, 1 out]
          n1224 = Build Array (concatenate)(w841, w835) -> (w842:dbl[])
          n1225 = local write "Numeric 3"(w822) -> ()
        }
        n1226 = local write "ROI Descriptor"(w504) -> ()
        n1227 = Unbundle(w547) -> ("X"=w546:i32)  [unwired: 1 out]
        n1228 = Add Array Elements(numeric array=w553) -> (sum=w564:dbl)
        n1229 = local write "Distances"(w553) -> ()
        n1230 = local write "Total Width"(w564) -> ()
        n1231 = local write "Zoom"(w546) -> ()
        n1232 = local read "Total Width"() -> (w507:dbl)
        n1233 = local read "Rec: Width"() -> (w505:dbl)
        n1234 = local read "Manual-Width"() -> (w503:bool)
        n1235 = Not(x=w503) -> (.not. x?=w501:bool)
        n1236 = Equal To 0?(x=w507) -> (x = 0?=w502:bool)
        n1237 = Or(x=w502, y=w503) -> (x .or. y?=w506:bool)
        n1238 = And(x=w502, y=w501) -> (x .and. y?=w500:bool)
        n1239 = case shown="True" w500 {
          tunnel: w505 -> [_ w582]
          frame False {
          }
          frame True {
            n1240 = local write "New: Width"(w582) -> ()
          }
        }
        n1241 = case shown="False" w506 {
          tunnel: w507 -> [w583 _]
          frame False {
            n1242 = local write "New: Width"(w583) -> ()
          }
          frame True {
          }
        }
        n1243 = local read "Manuel-Dielectric"() -> (w429:bool)
        n1244 = local read "Rec: Dielectric (d)"() -> (w428:dbl)
        n1245 = local read "Manuel-Length"() -> (w430:bool)
        n1246 = local read "Rec: Length"() -> (w431:dbl)
        n1247 = case shown="False" w430 {
          tunnel: w431 -> [w573 _]
          frame False {
            n1248 = local write "New: Length"(w573) -> ()
          }
          frame True {
          }
        }
        n1249 = case shown="False" w429 {
          tunnel: w428 -> [w572 _]
          frame False {
            n1250 = local write "New: Dielectric"(w572) -> ()
          }
          frame True {
          }
        }
      }
    }
  }
  n1251 = Build Array("DeviceID", "Fabricator", "Deposition", "Date", "Sample", "Row", "Column", "L (um)", "W (um)", "Material", "Treatment", "TC (mM)", "Solvent", "C (%)", "ST (C)", "Drops", "Wait (s)", "RT (F)", "RH (%)", "Ramp (s)", "RPM", "Accel (RPM/s)", "Time (s)", "Mobility", "On/Off", "Vt", "S.T.S") -> (→"Transformer \nHeaders":string[])
